vi "Master Control Loops Old.vi"() -> ()   [LabVIEW 2013]
uses:
  lib/DAQ IO/Daq Actions.ctl
  lib/Data Access Objects/Metadata/LBCB Number.ctl
  lib/Control Loop/Parameters Changes.ctl
  lib/Data Access Objects/Metadata/Persistant DAO Actions.ctl
  lib/MixedMode/Mixed Mode States.ctl
  lib/MixedMode/Ramp Time Tuple.ctl
  lib/MixedMode/Mixed Mode Command Action.ctl
  lib/MixedMode/Mixed Mode Convergence Status.ctl
  lib/MixedMode/Mixed Mode Cartesian Data.ctl
  lib/MixedMode/Target Data.ctl
  lib/MixedMode/Messages/Mixed Mode Command.ctl
  lib/Control Loop/Mixed Mode Hold Data type.ctl
  lib/Control Loop/Control Loop State.ctl
  lib/Data Access Objects/Metadata/DAO Actions.ctl
  lib/Control Loop/Parameter Change States.ctl
  lib/MixedMode/Messages/Mixed Mode Status.ctl
  lib/Apps/App Status Actions.ctl
  lib/Logging/LogFileType.ctl
  lib/Launcher/Launcher Actions.ctl
  lib/Launcher/NoPanelAppTypes.ctl
  lib/Autobalance/Autobalance State.ctl
  lib/Apps/Yes No Button.ctl
  lib/Control Loop/Limit Settings.ctl
  lib/Control Loop/Limit Matrix.ctl
  lib/Data Access Objects/Global Cache/Global Cache.vi
  lib/Control Loop/MM Result Actions.ctl
  lib/MixedMode/Stiffness Matrix.ctl
  lib/Limits/Cart Disp Faults.ctl
  lib/Limits/Cart Force Faults.ctl
  lib/Limits/Actuator Faults.ctl
  lib/Control Loop/Act & Cart Commands.ctl
  lib/Limits/Within Limits Matrix.ctl
  lib/Global Data/Jacobian Stiffness Column Id.ctl
  lib/Global Data/Jacobian Stiffness Column.ctl
  lib/Global Data/Dataset Source.ctl
  lib/Logging/Command or Stiffness Updates.ctl
  lib/Control Loop/Command Or Stiffness Update Type.ctl
  lib/Data Access Objects/Control Loop/PID Controls.ctl
  lib/Autobalance/Autobalance Status Data.ctl
  lib/Autobalance/Autobalance Stage.ctl
  lib/Autobalance/Autobalance Data Point.ctl
  lib/Control Loop/Measurements.ctl
  lib/Data Access Objects/Autobalance/Autobalance Control Parameters.ctl
panel:
  out "MM Result Actions":T1
  out "Commands":T2[](array[typedef])
  out "Stiffness Jacobian Column":T3[](array[typedef])
  out "Target":T5[](array[typedef])
  out "Cart Individual Cmds":dbl[][](array[numeric])=[[0.015224103858920254, 0.016374115079328375, 0.0001743188568230551, 0.03971045114557009, 0.007082336209989981, 0.009859079687370698, 8.685887933911959, 1.9897804119684945, 4.857688782335148, 93.30834661628205, -5.911514458784602, -1.446477360303783]]
  in  "AB Parameters":T6={"Number of Samples"=0, "Delay After Cmd"=0, "Maximum Command"=0.0, "1/4 Linear Range"=0.5}
  out "Increment Limits":T2[](array[typedef])
  out "Hold Data":T7[](array[typedef])
  in  "L2 Ctrl Loop In Actuator":dbl[](array[numeric])
  out "Rigid Connection":bool
  out "Stiffness Limits":dbl[][][](array[numeric])
  out "L2 Autobalance Out":T8[](array[typedef])
  out "L2 Cmd  Volts":dbl[](array[numeric])
  out "L2 Ctrl Loop Out Actuator":dbl[](array[numeric])=[0.012801822908652838, 0.012801822908652838, 7.98290599846041e-06, 8.154359441903125e-06, 8.154359441903125e-06, 8.154359441903125e-06]
  in  "Monitor Loop Time":u32
  in  "Volts LVDT & LC":dbl[][](array[numeric])
  out "L1 Autobalance Out":T8[](array[typedef])
  out "Collecting DAQ Samples":bool
  out "DAQ Volts":dbl[](array[numeric])=[-5.059315779335383, -5.016629198362524, -5.097891313865665, -5.092890991738198, -5.1138932889519, -4.974194835814303, 0.24442110332308561, 0.2508540081873783, -0.00045656932832031883, -0.0010919008583725697, -0.001119467422792373, -0.001138029771633142, 0.051584220664617125, 0.05637080163747566, -0.0007913138656640637, 0.023009008261802286, -0.021593288951899364, 0.0027051641856972383, -5.059665406563526, -5.018353952939143, -5.097893414204858, -5.0928919356893525, -5.11389113151188, -4.974191443340161, 0.24267296718237016, 0.2422302353042843, -0.0004670710242903981, -0.0011032282722249686, -0.0010935781425555466, -0.0010973200819313358, 0.05123459343647403, 0.05464604706085686, -0.0007934142048580796, 0.02300806431064792, -0.02159113151187963, 0.0027085566598390553, 0.048884220664617124, 0.04853459343647403, 0.050170801637475664, 0.04844604706085686, -9.131386566406377e-05, -9.341420485807962e-05]
  in  "Volt Logger Time":u32
  out "All Stopped":bool
  out "Previous Target":T12[](array[typedef])
  out "Iterative Target":T5[](array[typedef])
  out "Mixed Mode":i32
  out "Status Changes":i32
  out "L2 Control Rate":i32
  out "DAQ Started":bool
  out "Current Target":T5[](array[typedef])
  out "Logging Directory":path
  out "Auto Balance Error Tolerance":dbl[][](array[numeric])=[[0.01, 0.01, 0.01, 0.01, 0.01, 0.01]]
  in  "Hold Period":bool
  in  "Averaging":bool
  out "L1 Ctrl Loop State":T13
  out "Max Increment":dbl[][](array[numeric])
  out "Jacobian Gain":dbl[][](array[numeric])
  out "Force Error Range":dbl[][](array[numeric])
  in  "L2 PID On":bool
  in  "Limits Check":T14[](array[typedef])
  in  "Ramp Time":u32
  out "Limits":T18[](array[typedef])
  out "Measurements":T20[](array[typedef])
  out "Stiffness Jacobian":cluster{T21}[](array[cluster])
  out "Convergence Status":T22[](array[typedef])
  out "MixedModeStates":T23
  out "PID Control":T24[](array[typedef])
  in  "L1 PID On":bool
  out "LBCB 1 Control Loop Force Limit":bool
  out "L2 Ctrl Loop State":T13
  out "L1 Cmd  Volts":dbl[](array[numeric])
  out "L1 Ctrl Loop Out Actuator":dbl[](array[numeric])=[0.012801822908652838, 0.012801822908652838, 7.98290599846041e-06, 8.154359441903125e-06, 8.154359441903125e-06, 8.154359441903125e-06]
  out "L1 Control Rate":i32=50 caption="Control Rate"
  in  "L1 Ctrl Loop In Actuator":dbl[](array[numeric])
  out "Number of \nExternal \nChannels":i32
  out "DAQ Enabled":bool
  in  "App Running":bool
  out "DAQ Rate":i32=2 caption="Control Rate"
  out "Servo Error":dbl[][](array[numeric])=[[-0.014471871278962644, -0.0027477897622864888, 0.03594582291831433, -0.006177356244415369, -0.000527948512754489, 0.04718526152757189]]
  out "Actuator Meas. Disp & Forces":dbl[][](array[numeric])=[[0.015224103858920254, 0.016374115079328375, 0.0001743188568230551, 0.03971045114557009, 0.007082336209989981, 0.009859079687370698, 8.685887933911959, 1.9897804119684945, 4.857688782335148, 93.30834661628205, -5.911514458784602, -1.446477360303783]]
  out "External Sensors":dbl[](array[numeric])
  out "DAQ Overflow":bool
  # "(Volts)"
  # "Cmd"
  # "Servo"
  # "Cmd"
  # "Servo"
  # "Cmd"
  # "Servo"
  # "Cmd"
  # "Servo"
  # "Continuous"
  # "Hold"
types:
  T1 = typedef "MM Result Actions.ctl" = enum16{"Nop", "Set Command", "Check Limits", "Send Command", "Store Prev Reading", "Averaging On", "Averaging Off", "Hold On", "Hold Off", "PID Hold On", "PID Hold Off", "Clear Increment Faults", "Set Initial Position"}
  T2 = typedef "Act & Cart Commands.ctl" = cluster{"Act Cmd":dbl[], "Cart Cmd":dbl[]}
  T3 = typedef "Jacobian Stiffness Column.ctl" = cluster{"Id":T4, "Column":dbl[]}
  T4 = typedef "Jacobian Stiffness Column Id.ctl" = enum16{"dDx", "dDy", "dDz", "dRx", "dRy", "dRz"}
  T5 = typedef "Target Data.ctl" = cluster{"Displacements":dbl[], "Command Type":enum16{"<None>", "Displacement", "Force"}[], "Forces":dbl[]}
  T6 = typedef "Autobalance Control Parameters.ctl" = cluster{"Number of Samples":i32, "Delay After Cmd":i32, "Maximum Command":dbl, "1/4 Linear Range":dbl}
  T7 = typedef "Mixed Mode Hold Data type.ctl" = cluster{"Displacements":dbl[], "Forces":dbl[], "Displacement \nCommands":dbl[]}
  T8 = typedef "Autobalance Status Data.ctl" = cluster{"IsBalanced":T9, "Autobalance Stage":T10, "High":T11, "Low":T11, "Balanced \nCmd":dbl}
  T9 = typedef "Yes No Button.ctl" = bool
  T10 = typedef "Autobalance Stage.ctl" = enum16{"Coarse", "Fine", "Backing Up", "Done"}
  T11 = typedef "Autobalance Data Point.ctl" = cluster{"cCmd":dbl, "cServo":dbl, "pCmd":dbl, "pServo":dbl}
  T12 = typedef "Mixed Mode Cartesian Data.ctl" = cluster{"Displacements":dbl[], "Forces":dbl[]}
  T13 = typedef "Control Loop State.ctl" = enum16{"Idle", "Off", "Reset Autobalancing", "Autobalancing", "Set Command", "Ready for Control", "On"}
  T14 = typedef "Within Limits Matrix.ctl" = cluster{"Act Disp":T15, "Act Force":T15, "Act Incr":T15, "Cart Disp":T16, "Cart Force":T17, "Cart Incr":T16}
  T15 = typedef "Actuator Faults.ctl" = cluster{"X1":bool, "X2":bool, "Y1":bool, "Z1":bool, "Z2":bool, "Z3":bool}
  T16 = typedef "Cart Disp Faults.ctl" = cluster{"Dx":bool, "Dy":bool, "Dz":bool, "Rx":bool, "Ry":bool, "Rz":bool}
  T17 = typedef "Cart Force Faults.ctl" = cluster{"Fx":bool, "Fy":bool, "Fz":bool, "Mx":bool, "My":bool, "Mz":bool}
  T18 = typedef "Limit Settings.ctl" = cluster{"Actuator Force Limits":T19, "Actuator Stroke Limits":T19, "Cartesian Disp Limit":T19, "Cartesian Force Limit":T19}
  T19 = typedef "Limit Matrix.ctl" = dbl[][]
  T20 = typedef "Measurements.ctl" = cluster{"Act Disp":dbl[], "Act Forces":dbl[], "Cart Disp":dbl[], "Cart Forces":dbl[]}
  T21 = typedef "Stiffness Matrix.ctl" = dbl[][]
  T22 = typedef "Mixed Mode Convergence Status.ctl" = cluster{"IsConverged":bool[], "Force Errors":dbl[], "Controlling DOF":bool[]}
  T23 = typedef "Mixed Mode States.ctl" = enum16{"Init", "Wait For DAQ", "Idle", "Start Initial Position", "Initial Position", "Start Initial Ramp", "Run Initial Ramp", "Start Iterative Stage", "Convergence Check", "Update Stiffness Jacobian", "Update Command", "Start Iterative Ramp", "Run Iterative Ramp", "Start Iterative Stabilize", "Iterative Stabilize", "Start Iterative Holding", "Iterative Holding", "Start Stabilize", "Stabilize", "Start Hold", "Holding", "Done", "Aborting", "Exit", "Nop"}
  T24 = typedef "PID Controls.ctl" = cluster{"I-Control":bool, "Ctrl Mode":bool}
  T25 = typedef "Command Or Stiffness Update Type.ctl" = cluster{"Target":T5[], "Stiffness":T3[], "Command || Stiffness Update":T26}
  T26 = typedef "Command or Stiffness Updates.ctl" = enum16{"Command Update", "Iterative Command Update", "Stiffness Update"}
  T27 = cluster{"Act Disp":dbl[], "Act Forces":dbl[], "Cart Disp":dbl[], "Cart Forces":dbl[]}
  T28 = typedef "LBCB Number.ctl" = enum16{"LBCB1", "LBCB2"}
  T29 = typedef "Persistant DAO Actions.ctl" = enum16{"Init", "Get", "Set", "Load", "Save"}
  T30 = typedef "Autobalance State.ctl" = enum16{"Init", "Send High ", "Wait High", "Read High Start", "Read High", "Send Low", "Wait Low", "Read Low Start", "Read Low", "Publish", "Calculate", "Done"}
  T31 = typedef "Ramp Time Tuple.ctl" = cluster{"Ramp":dbl, "Stab":dbl, "Hold":dbl}
  T32 = typedef "Mixed Mode Command Action.ctl" = enum16{"Start Command", "Stop", "Exit", "No Op", "Start Acquisition", "Measure Initial Position"}
  T33 = typedef "Mixed Mode Status.ctl" = cluster{"LBCB Target":T5[], "MixedModeStates":T23, "LBCB Convergence":T22[], "LBCB Measurements":T12[]}
  T34 = typedef "Mixed Mode Command.ctl" = cluster{"Command":T32, "Ramp Times":cluster{"Initial":T31, "Iterative":T31}, "LBCB1":T5, "LBCB2":T5}
  T35 = typedef "Parameters Changes.ctl" = cluster{"Change State":T36, "LBCB Number":T28}
  T36 = typedef "Parameter Change States.ctl" = enum16{"Mixed Mode", "Control Loop", "Limits", "Application", "Stiffness Jacobian", "Start DAQ", "Reset Auto-Balance", "Set Command", "Enable Control", "Disable Control", "Position", "Stop Application"}
  T37 = typedef "DAO Actions.ctl" = enum16{"Init", "Get", "Set"}
  T38 = typedef "Number Of LBCBs.ctl" = enum16{"1", "2"}
  T39 = typedef "Cartesian Point.ctl" = cluster{"Dx":dbl, "Dy":dbl, "Dz":dbl, "Rx":dbl, "Ry":dbl, "Rz":dbl}
  T40 = typedef "Actuator Matrix.ctl" = cluster{"Lower":T41, "Upper":T41}
  T41 = typedef "Actuator Point.ctl" = cluster{"X1":dbl, "X2":dbl, "Y1":dbl, "Z1":dbl, "Z2":dbl, "Z3":dbl}
  T42 = typedef "Cartesian Matrix.ctl" = cluster{"Lower":T39, "Upper":T39}
  T43 = typedef "App Parameters.ctl" = cluster{"Monitor Loop":T44, "Ramp Time":T44, "Log Loop":T44, "TCP to DAQ":T44, "Logging Directory":path, "Log File Size (MBytes)":i64, "Volt Logging Loop":T44, "2 LBCB Archiving Mode":bool, "Fake":bool}
  T44 = typedef "Timing Parameters.ctl" = cluster{"Interval":dbl, "Rate ":dbl}
  T45 = typedef "Dataset Source.ctl" = enum16{"Continuous", "Hold", "ED", "Volts", "Offsets", "Increments"}
  T46 = typedef "Calibration Settings.ctl" = cluster{"Command Sensitivity":dbl[], "Servo Error Offset":dbl[], "LVDT Sensitivity":dbl[], "LVDT Offset":dbl[], "Load Cell Offsets":dbl[], "Load Cell Sensitivity":dbl[]}
  T47 = typedef "App Status Actions.ctl" = enum16{"Init", "Get Status", "Running", "Control", "Autobalanced", "Data Acquisition", "Set App State", "DAQ Started", "Set LBCB State", "Set All", "Set Cont Logging", "Set Step Logging", "Set MM Logging", "Set Volt Logging", "Set DAQ Link"}
  T48 = typedef "Force Control Parameters.ctl" = cluster{"Use Force Error Range Ratios":bool, "Use Group Priorities":bool, "Multi Command Update":bool, "Steps per Stiffness \nMeasurement":i32}
  T49 = typedef "Cartesian Force Vector.ctl" = cluster{"Fx":dbl, "Fy":dbl, "Fz":dbl, "Mx":dbl, "My":dbl, "Mz":dbl}
  T50 = typedef "Ramp Time Input.ctl" = cluster{"Directional":T51, "Iterative":T51}
  T51 = typedef "Ramp Control.ctl" = cluster{"Ramp":dbl, "Stabilize":dbl, "Hold":dbl}
  T52 = typedef "App Status.ctl" = cluster{"Running":bool, "Controlling L2":bool, "Autobalance L2":bool, "Data Acquisition":bool, " App State":T53, "DAQ Started":bool, "LBCB 1 State":T54, "LBCB 2 State":T54, "Controlling L1":bool, "Autobalance L1":bool, "Continuous Logging":bool, "Step Logging":bool, "Voltage Logging":bool, "Mixed Mode Logging":bool, "DAQ Link":bool}
  T53 = typedef "AppStates.ctl" = enum16{"Starting OM", "Initializing Displays", "Setting up Archiving", "Setting Up DAQ Channels", "Start DAQ", "DAQ Starting", "Controlling LBCBs", "Stopping OM"}
  T54 = typedef "Lbcb Control Loop States.ctl" = enum16{"Idle", "Start Selected", "Load Last Command", "Start Autobalancing", "Autobalancing", "Control Loop Initialized", "Control Enabled"}
  T55 = cluster{"Act Disp":dbl[], "Act Forces":dbl[], "Cart Disp":dbl[], "Cart Forces":dbl[]}[]
  T56 = typedef "Daq Actions.ctl" = enum16{"Init", "Send Commands", "Get Responses", "Stop"}
  T57 = enum16{"open", "replace", "create", "open or create", "replace or create", "replace or create with confirmation"}
  T58 = typedef "LogFileType.ctl" = enum16{"Continuous", "Step", "Volts", "Offsets", "DLL  Errors", "Snapshot", "Commands", "StiffnessUpdates", "Debug", "End List"}
  T59 = typedef "NoPanelAppTypes.ctl" = enum16{"NTCP Socket", "Data Archiving", "DAQ Link", "Control Loops", "Cmd Disp Diffs", "LBCB Data", "Limits", "Mixed Mode Widget", "Offsets", "Debug"}
  T60 = typedef "Launcher Actions.ctl" = enum16{"Launch", "Stop All", "Stop", "Kill", "Running?", "Init"}
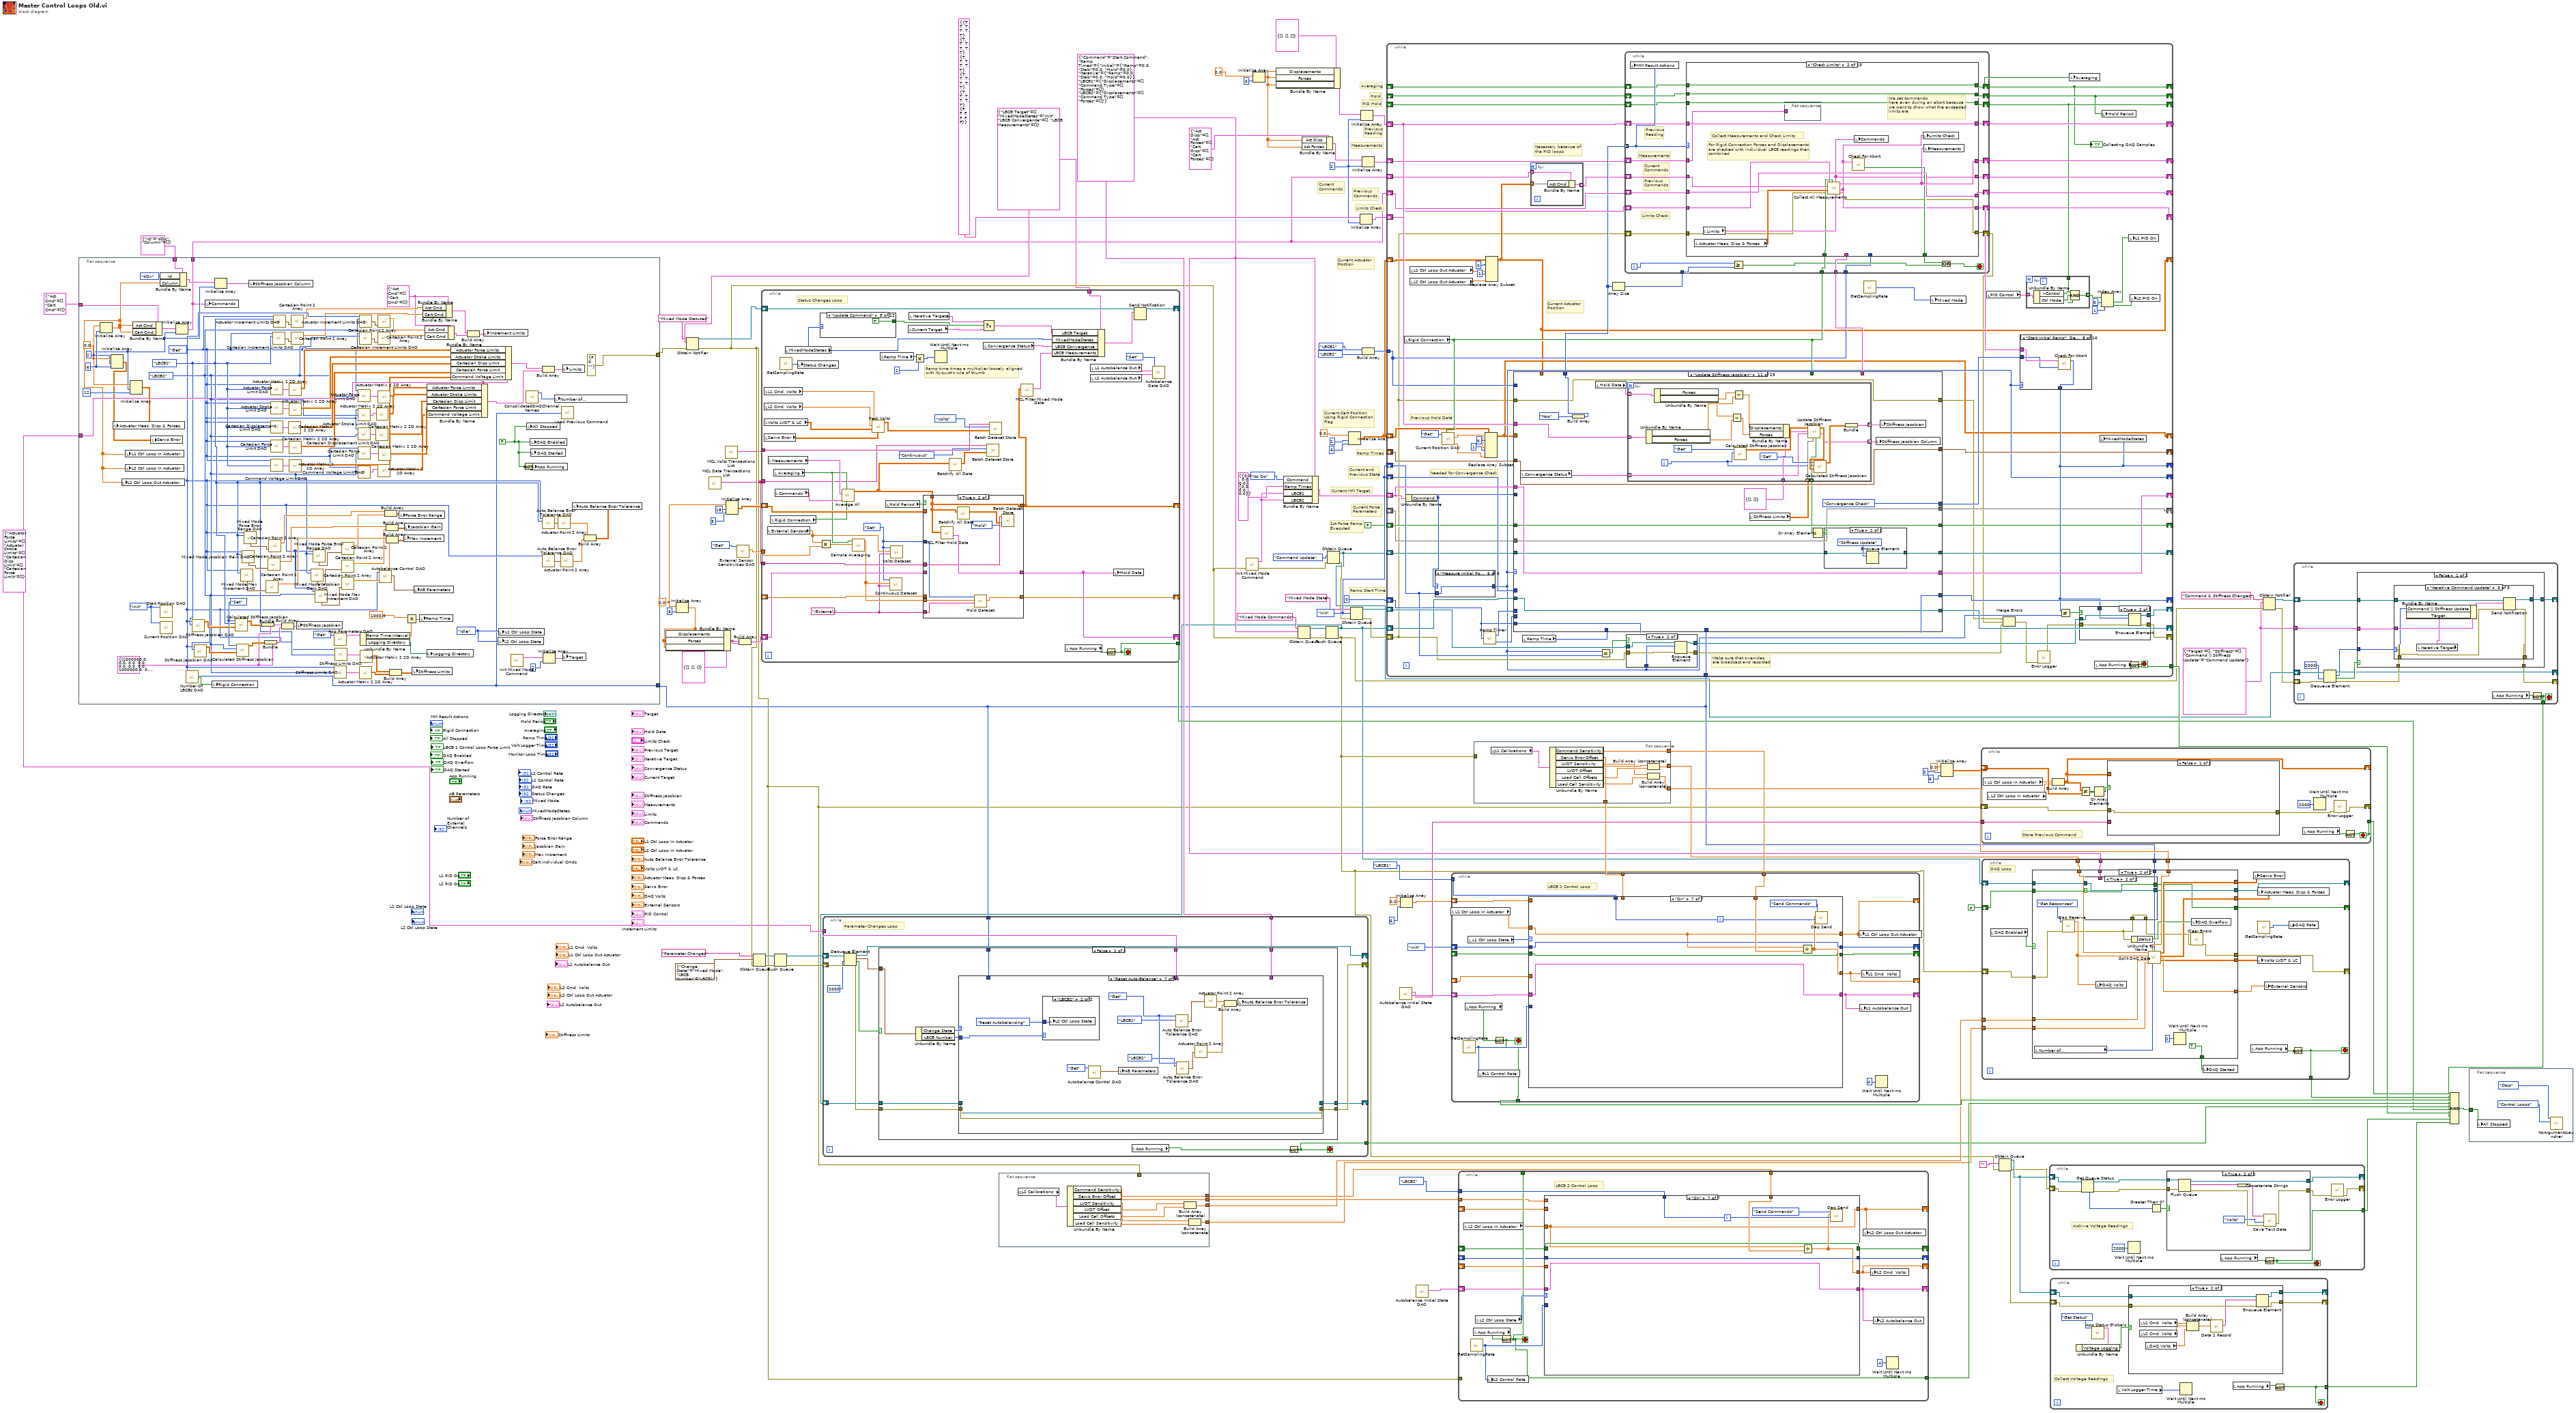
[diagram p0: block diagram]
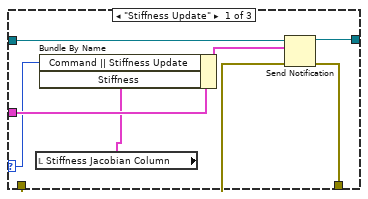
[diagram p2: hidden frame]
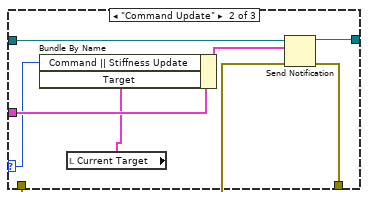
[diagram p3: hidden frame]
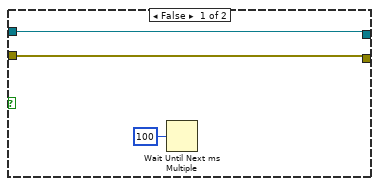
[diagram p5: hidden frame]
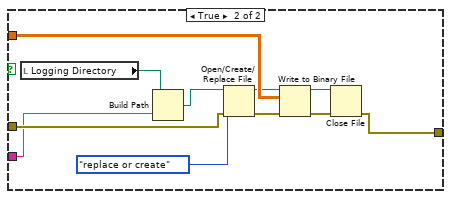
[diagram p7: hidden frame]
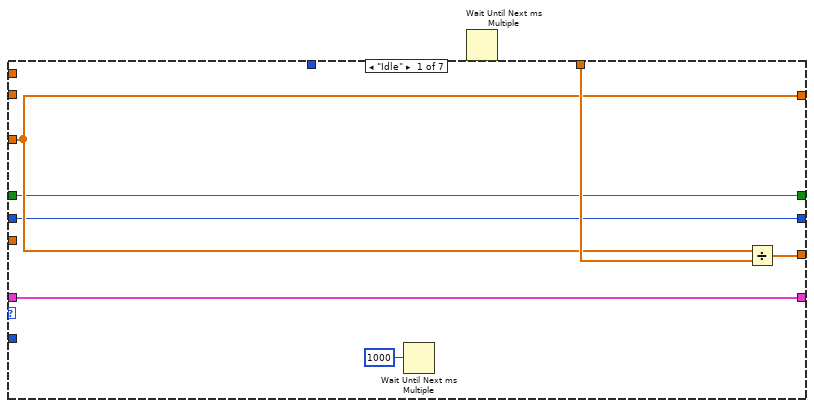
[diagram p8: hidden frame]
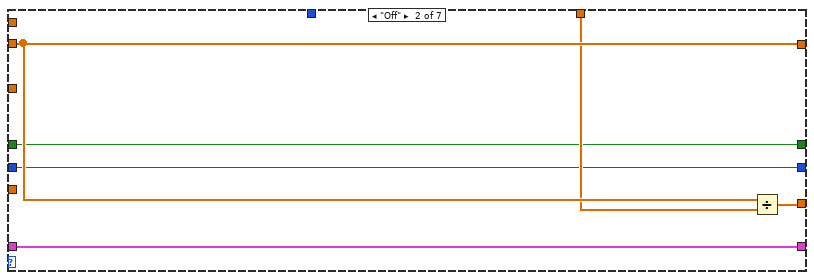
[diagram p9: hidden frame]
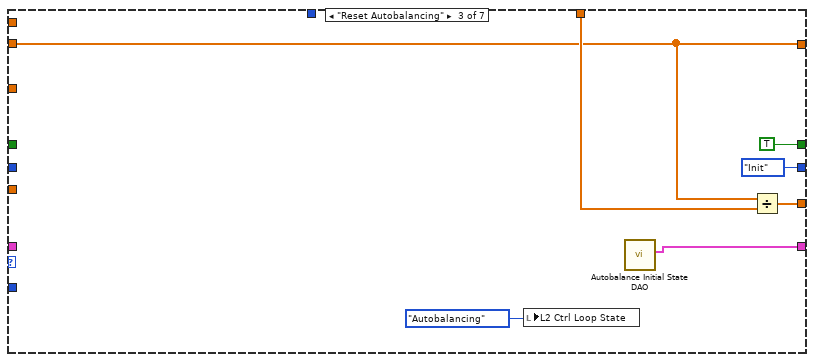
[diagram p10: hidden frame]
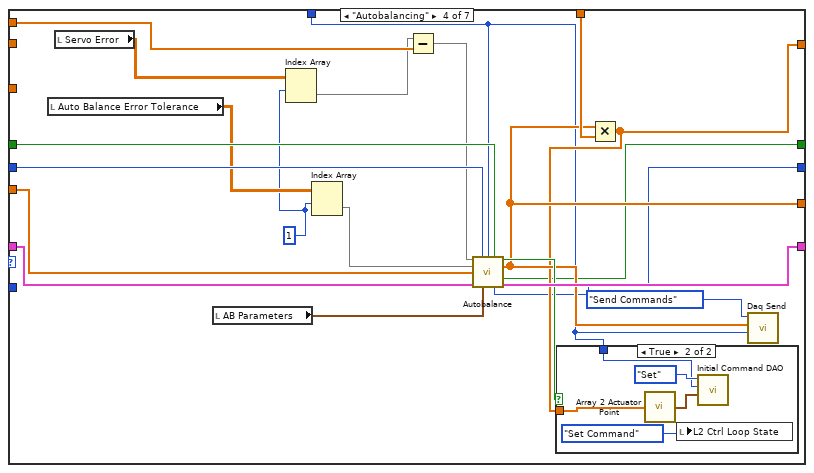
[diagram p11: hidden frame]
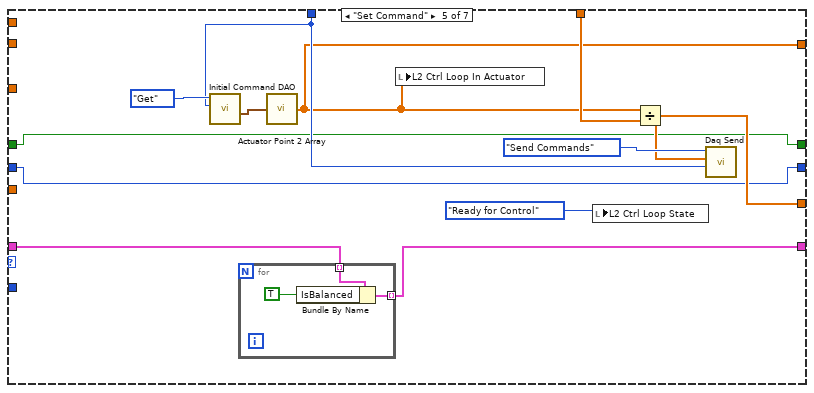
[diagram p13: hidden frame]
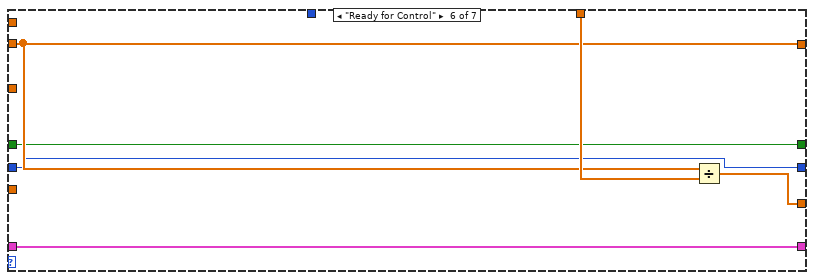
[diagram p14: hidden frame]
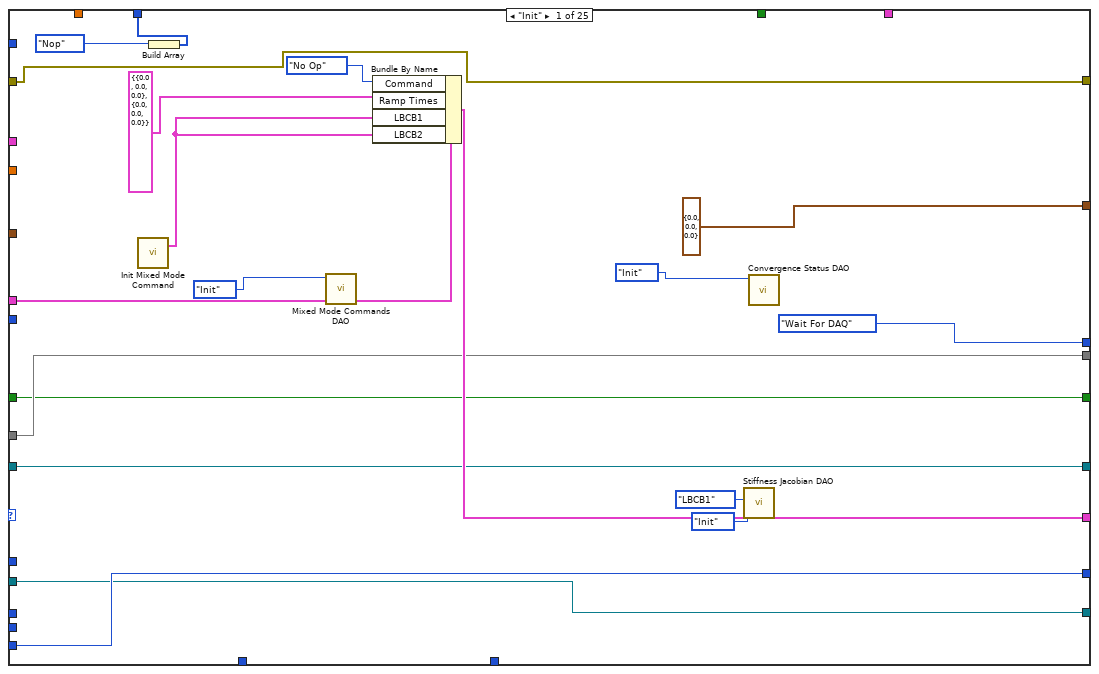
[diagram p15: hidden frame]
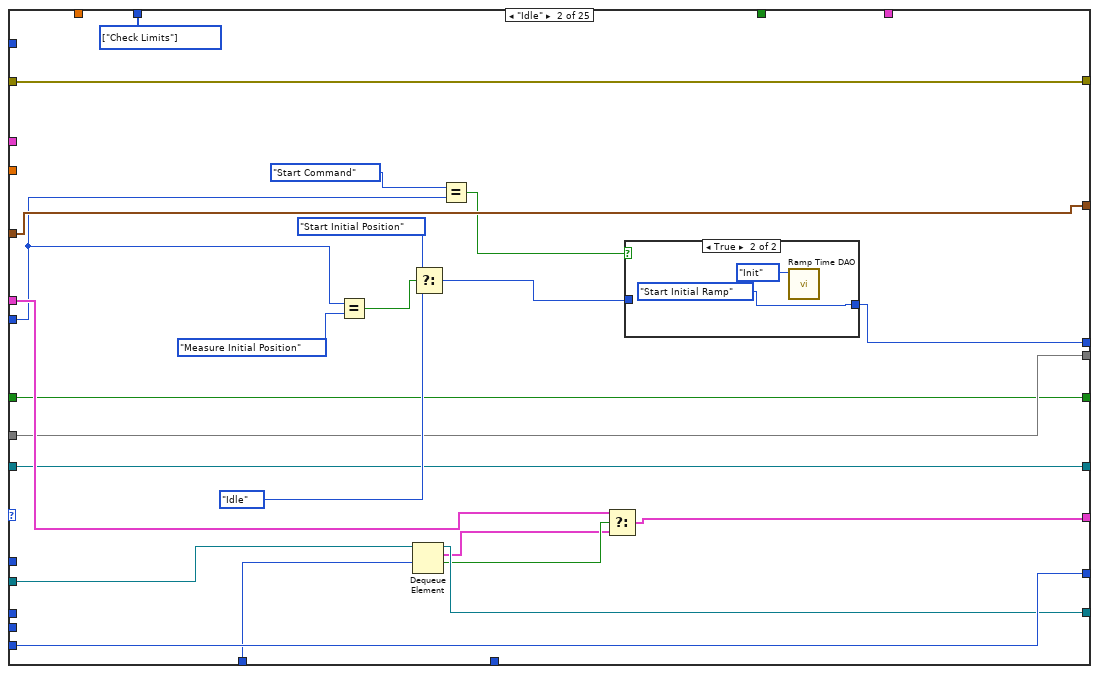
[diagram p16: hidden frame]
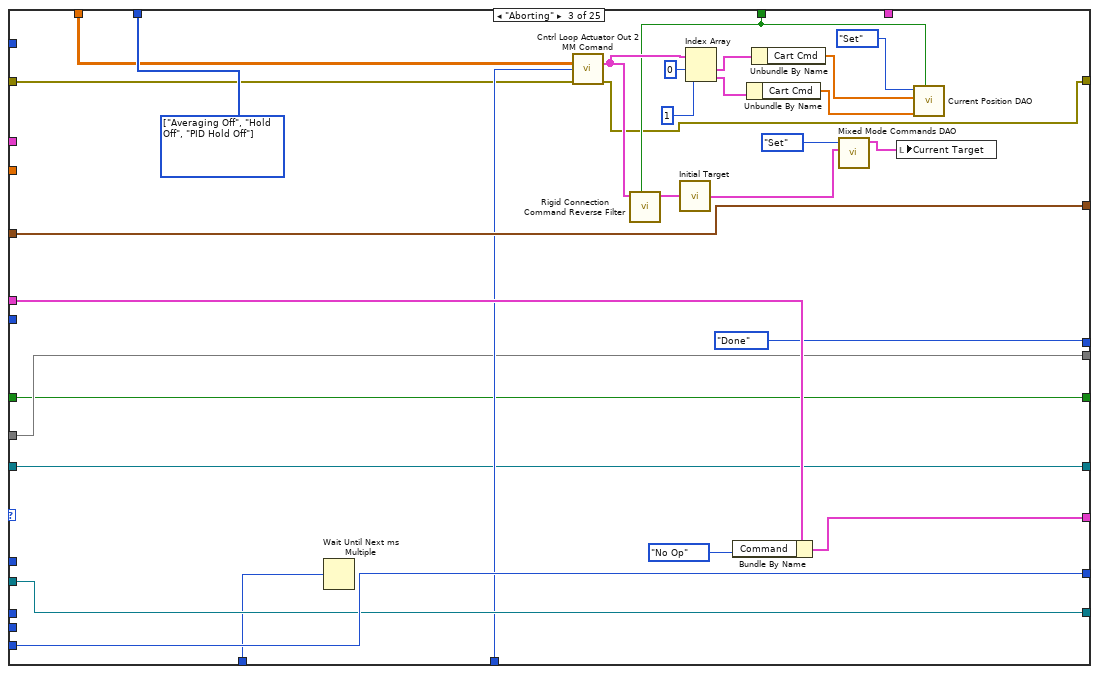
[diagram p18: hidden frame]
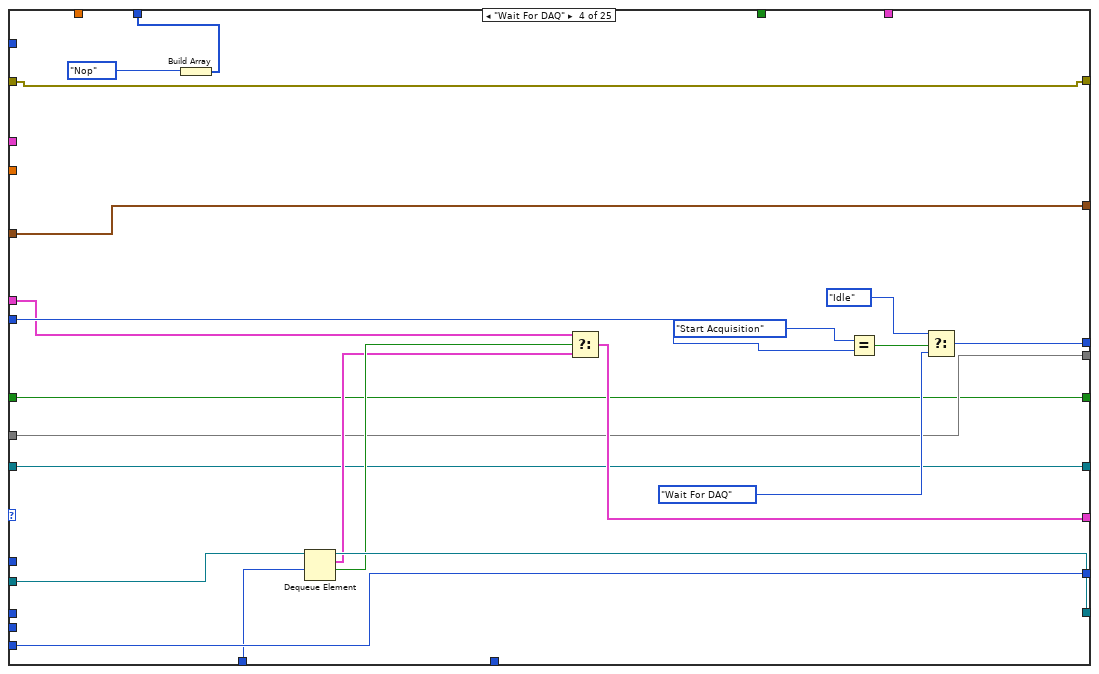
[diagram p19: hidden frame]
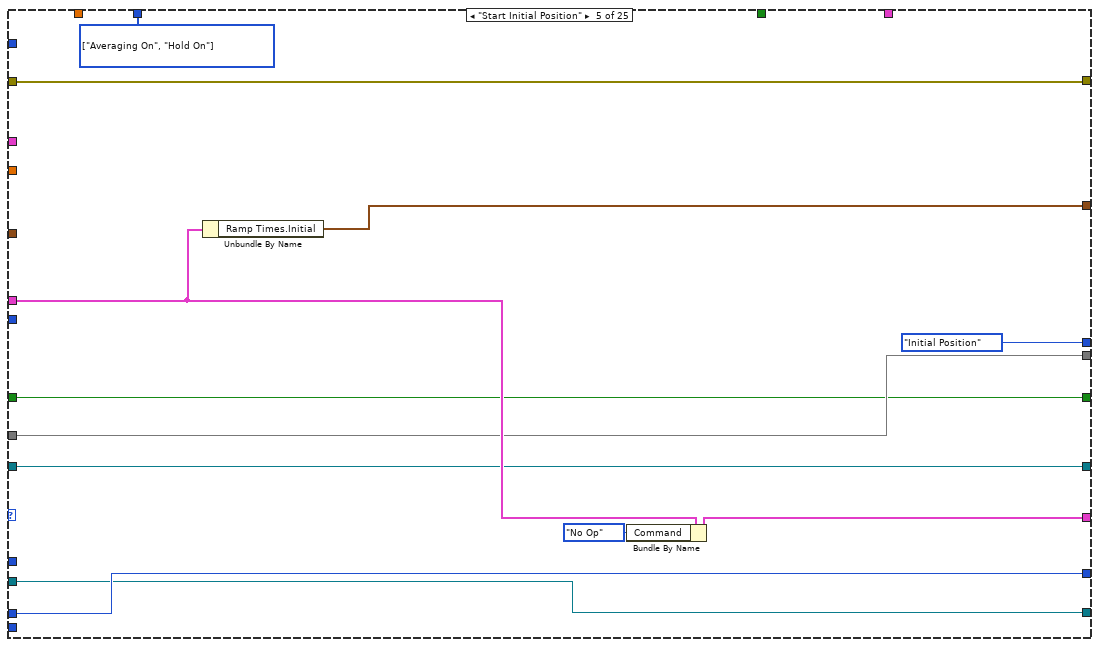
[diagram p20: hidden frame]
diagram:
  w7 = T25 {"Target"=[], "Stiffness"=[], "Command || Stiffness Update"=enum."Command Update"} ("Command || Stiffness Update")
  w18 = 0.0 ("element")
  w38 = 2 ("dimension size")
  w59 = T18 {"Actuator Force Limits"=[], "Actuator Stroke Limits"=[], "Cartesian Disp Limit"=[], "Cartesian Force Limit"=[]} ("L1  Limits")
  w97 = T33 {"LBCB Target"=[], "MixedModeStates"=enum."Init", "LBCB Convergence"=[], "LBCB Measurements"=[]} ("Mixed Mode Status")
  w57 = T34 {"Command"=enum."Start Command", "Ramp Times"={"Initial"={"Ramp"=0.0, "Stab"=0.0, "Hold"=0.0}, "Iterative"={"Ramp"=0.0, "Stab"=0.0, "Hold"=0.0}}, "LBCB1"={"Displacements"=[], "Command Type"=[], "Forces"=[]}, "LBCB2"={"Displacements"=[], "Command Type"=[], "Forces"=[]}} ("Mixed Mode Command")
  w104 = Mixed_Mode_States."Init" ("MixedModeStates")
  # "Current Actuator\nPostion"
  # "Current Cart Position\nUsing Rigid Connection\nFlag"
  # "1st Force Ramp\nExecuted"
  # "Current Force\nParameters"
  # "Previous\nCommands"
  # "Limits Check"
  # "Ramp Start Time"
  # "PID Hold"
  # "Hold"
  # "Averaging"
  # "Previous\nReading"
  # "Current \nCommands"
  # "Measurements"
  # "Current MM Target"
  # "Current and\nPrevious State"
  # "Ramp Times"
  n1 = flat-sequence {
    tunnel: [errorcluster {"status"=FALSE, "code"=0, "source"=""} ("error out")] -> w62
    tunnel: w59 -> [w188]
    tunnel: [w109] -> w39
    tunnel: [w112] -> w37
    tunnel: T3 {"Id"=enum."dDx", "Column"=[]} ("Jacobian Stiffness Column") -> [w121]
    tunnel: T2 {"Act Cmd"=[], "Cart Cmd"=[]} ("Data") -> [w116]
    frame #0 {
      w123 = DAO_Actions."Init" ("DAO Actions")
      w125 = T2 {"Act Cmd"=[], "Cart Cmd"=[]} ("Data")
      w156 = cluster{T21} {[[1000000.0, 0.0, 0.0, 0.0, 0.0, 0.0], [0.0, 1000000.0, 0.0, 0.0, 0.0, 0.0], [0.0, 0.0, 1000000.0, 0.0, 0.0, 0.0], [0.0, 0.0, 0.0, 1000000.0, 0.0, 0.0], [0.0, 0.0, 0.0, 0.0, 1000000.0, 0.0], [0.0, 0.0, 0.0, 0.0, 0.0, 1000000.0]]} ("Cluster")
      w122 = 2 ("dimension size")
      w190 = Control_Loop_State."Idle" ("L1 Ctrl Loop State")
      w160 = 6 ("dimension size")
      w159 = 0.0 ("element")
      w133 = LBCB_Number."LBCB2" ("ID")
      w134 = LBCB_Number."LBCB1" ("ID")
      w132 = Persistant_DAO_Actions."Get" ("Actuator Force Limit Actions")
      w194 = FALSE
      w200 = Persistant_DAO_Actions."Set" ("Actions")
      n2 = Initialize Array(w159, w160) -> (w119:dbl[])
      n3 = Initialize Array(w159, w122, w160) -> (w137:dbl[][])
      n4 = local write "L1 Ctrl Loop Out Actuator"(w119) -> ()
      n5 = local write "L1 Ctrl Loop In Actuator"(w119) -> ()
      n6 = local write "L2 Ctrl Loop In Actuator"(w119) -> ()
      n7 = Initialize Array(w159, w122, 12 ("dimension size")) -> (w124:dbl[][])
      n8 = local write "Actuator Meas. Disp & Forces"(w124) -> ()
      n9 = Bundle By Name(cluster=w116, "Act Cmd"=w119, "Cart Cmd"=w119) -> (w142:T2)
      n10 = local write "Servo Error"(w137) -> ()
      n11 = call "Start Position DAO.vi"("DAO Actions"=w123) -> ()  [unwired: 9 in, 2 out]
      n12 = call "Current Position DAO.vi"("Actions"=w123) -> ()  [unwired: 9 in, 2 out]
      n13 = Bundle By Name(cluster=w121, "Id"=Jacobian_Stiffness_Column_Id."dDx", "Column"=w119) -> (w118:T3)
      n14 = Initialize Array(w142, w122) -> (w112:T2[])
      n15 = call "Number Of LBCBs DAO.vi"("Actions"=w132) -> ("Number of\nLBCBs Out"=w109:T38, "Rigid Connection Out"=w143:bool)  [unwired: 13 in, 4 out]
      n16 = call "Stiffness Jacobian DAO.vi"("LBCB Number"=w134, "Actions"=w132) -> ("Stiffness Jacobian Out"=w199:T21)  [unwired: 3 in, 6 out]
      n17 = call "Stiffness Jacobian DAO.vi"("LBCB Number"=w133, "Actions"=w132) -> ("Stiffness Jacobian Out"=w201:T21)  [unwired: 3 in, 6 out]
      n18 = local write "Commands"(w112) -> ()
      n19 = local write "Rigid Connection"(w143) -> ()
      n20 = Initialize Array(w118, w122) -> (w117:T3[])
      n21 = call "Calculated Stiffness Jacobian.vi"("Stiffness Jacobian In"=w199, "LBCB Number"=w134, "Actions"=w200) -> ("Stiffness Jacobian Out"=w158:T21)  [unwired: 1 in, 7 out]
      n22 = call "Calculated Stiffness Jacobian.vi"("Stiffness Jacobian In"=w201, "LBCB Number"=w133, "Actions"=w200) -> ("Stiffness Jacobian Out"=w157:T21)  [unwired: 1 in, 7 out]
      n23 = call "Mixed Mode Max Increment DAO.vi"("Max Increment Actions"=w132, "LBCB Number"=w134) -> ("Max Increment Out"=w207:T39)  [unwired: 3 in, 10 out]
      n24 = call "Mixed Mode Jacobian Gain DAO.vi"("Jacobian Gain Actions"=w132, "LBCB Number"=w134) -> ("Jacobian Gain Out"=w206:T39)  [unwired: 3 in, 10 out]
      n25 = call "Mixed Mode Force Error Range DAO.vi"("Force Error Range Actions"=w132, "LBCB Number"=w134) -> ("Force Error Range Out"=w205:T39)  [unwired: 3 in, 10 out]
      n26 = local write "Stiffness Jacobian Column"(w117) -> ()
      n27 = Bundle(cluster=w156, w158) -> (w155:cluster{T21})
      n28 = Bundle(cluster=w156, w157) -> (w154:cluster{T21})
      n29 = call "Cartesian Point 2 Array.vi"("Cart Disp"=w207) -> ("Array"=w202:dbl[])  [unwired: 2 out]
      n30 = call "Cartesian Point 2 Array.vi"("Cart Disp"=w206) -> ("Array"=w203:dbl[])  [unwired: 2 out]
      n31 = call "Cartesian Point 2 Array.vi"("Cart Disp"=w205) -> ("Array"=w204:dbl[])  [unwired: 2 out]
      n32 = call "Actuator Force Limit DAO.vi"("Actuator Force Limit Actions"=w132, "ID"=w134) -> ("Actuator Force Limits Out"=w187:T40)  [unwired: 3 in, 10 out]
      n33 = call "Actuator Stroke Limit DAO.vi"("Actuator Stroke Limit Actions"=w132, "ID"=w134) -> ("Actuator Stroke Limits Out"=w186:T40)  [unwired: 3 in, 10 out]
      n34 = call "Cartesian Displacement Limit DAO.vi"("Cartesian Displacement Limit Actions"=w132, "ID"=w134) -> ("Cartesian Displacement Out"=w181:T42)  [unwired: 3 in, 10 out]
      n35 = call "Cartesian Force Limit DAO.vi"("Cartesian Force Limit Actions"=w132, "ID"=w134) -> ("Cartesian Force Limit Out"=w180:T42)  [unwired: 3 in, 10 out]
      n36 = call "Command Voltage Limit DAO.vi"("Actuator Stroke Limit Actions"=w132, "ID"=w134) -> ("Command Voltage Limit Out"=w185:T40)  [unwired: 3 in, 10 out]
      n37 = call "Cartesian Increment Limits DAO.vi"("Actions"=w132, "LBCB Number"=w134) -> ("Inc Limits Out"=w141:T39)  [unwired: 11 in, 2 out]
      n38 = call "Actuator Increment Limits DAO.vi"("Actions"=w132, "LBCB Number"=w134) -> ("Inc Limits Out"=w136:T41)  [unwired: 11 in, 2 out]
      n39 = Build Array(w155, w154) -> (w153:cluster{T21}[])
      n40 = call "Cartesian Matrix 2 2D Array.vi"("Matrix In"=w181) -> ("Matrix Out"=w169:T19)  [unwired: 10 out]
      n41 = call "Actuator Matrix 2 2D Array.vi"("Matrix In"=w187) -> ("Matrix Out"=w184:T19)  [unwired: 10 out]
      n42 = call "Actuator Matrix 2 2D Array.vi"("Matrix In"=w186) -> ("Matrix Out"=w183:T19)  [unwired: 10 out]
      n43 = call "Cartesian Matrix 2 2D Array.vi"("Matrix In"=w180) -> ("Matrix Out"=w168:T19)  [unwired: 10 out]
      n44 = call "Actuator Matrix 2 2D Array.vi"("Matrix In"=w185) -> ("Matrix Out"=w182:T19)  [unwired: 10 out]
      n45 = call "Cartesian Point 2 Array.vi"("Cart Disp"=w141) -> ("Array"=w129:dbl[])  [unwired: 2 in]
      n46 = call "Cartesian Point 2 Array.vi"("Cart Disp"=w136) -> ("Array"=w131:dbl[])  [unwired: 2 in]
      n47 = local write "Stiffness Jacobian"(w153) -> ()
      n48 = call "Mixed Mode Jacobian Gain DAO.vi"("Jacobian Gain Actions"=w132, "LBCB Number"=w133) -> ("Jacobian Gain Out"=w192:T39)  [unwired: 3 in, 10 out]
      n49 = call "Mixed Mode Force Error Range DAO.vi"("Force Error Range Actions"=w132, "LBCB Number"=w133) -> ("Force Error Range Out"=w191:T39)  [unwired: 3 in, 10 out]
      n50 = call "Mixed Mode Max Increment DAO.vi"("Max Increment Actions"=w132, "LBCB Number"=w133) -> ("Max Increment Out"=w193:T39)  [unwired: 3 in, 10 out]
      n51 = call "App Parameters DAO.vi"("Actions"=Persistant_DAO_Actions."Get") -> ("Application Timing and Logging Out"=w211:T43)  [unwired: 3 in, 7 out]
      n52 = call "Stiffness Limits DAO.vi"("Actions"=w132, "ID"=w133) -> ("Stiffness Limit Out"=w146:T42)  [unwired: 11 in, 2 out]
      n53 = call "Stiffness Limits DAO.vi"("Actions"=w132, "ID"=w134) -> ("Stiffness Limit Out"=w148:T42)  [unwired: 11 in, 2 out]
      n54 = call "Cartesian Point 2 Array.vi"("Cart Disp"=w191) -> ("Array"=w166:dbl[])  [unwired: 1 in, 1 out]
      n55 = call "Cartesian Point 2 Array.vi"("Cart Disp"=w192) -> ("Array"=w164:dbl[])  [unwired: 1 in, 1 out]
      n56 = call "Cartesian Point 2 Array.vi"("Cart Disp"=w193) -> ("Array"=w162:dbl[])  [unwired: 1 in, 1 out]
      n57 = call "Actuator Force Limit DAO.vi"("Actuator Force Limit Actions"=w132, "ID"=w133) -> ("Actuator Force Limits Out"=w179:T40)  [unwired: 3 in, 10 out]
      n58 = call "Actuator Stroke Limit DAO.vi"("Actuator Stroke Limit Actions"=w132, "ID"=w133) -> ("Actuator Stroke Limits Out"=w178:T40)  [unwired: 3 in, 10 out]
      n59 = call "Cartesian Displacement Limit DAO.vi"("Cartesian Displacement Limit Actions"=w132, "ID"=w133) -> ("Cartesian Displacement Out"=w177:T42)  [unwired: 3 in, 10 out]
      n60 = call "Cartesian Force Limit DAO.vi"("Cartesian Force Limit Actions"=w132, "ID"=w133) -> ("Cartesian Force Limit Out"=w176:T42)  [unwired: 3 in, 10 out]
      n61 = call "Command Voltage Limit DAO.vi"("Actuator Stroke Limit Actions"=w132, "ID"=w133) -> ("Command Voltage Limit Out"=w175:T40)  [unwired: 3 in, 10 out]
      n62 = call "Cartesian Increment Limits DAO.vi"("Actions"=w132, "LBCB Number"=w133) -> ("Inc Limits Out"=w140:T39)  [unwired: 11 in, 2 out]
      n63 = call "Actuator Increment Limits DAO.vi"("Actions"=w132, "LBCB Number"=w133) -> ("Inc Limits Out"=w135:T41)  [unwired: 11 in, 2 out]
      n64 = call "Actuator Matrix 2 2D Array.vi"("Matrix In"=w146) -> ("Matrix Out"=w145:T19)  [unwired: 10 out]
      n65 = Unbundle By Name(w211) -> ("Ramp Time.Interval"=w212:dbl, "Logging Directory"=w208:path)
      n66 = call "Actuator Matrix 2 2D Array.vi"("Matrix In"=w148) -> ("Matrix Out"=w147:T19)  [unwired: 10 out]
      n67 = call "Cartesian Matrix 2 2D Array.vi"("Matrix In"=w177) -> ("Matrix Out"=w172:T19)  [unwired: 10 out]
      n68 = call "Actuator Matrix 2 2D Array.vi"("Matrix In"=w178) -> ("Matrix Out"=w173:T19)  [unwired: 10 out]
      n69 = call "Cartesian Point 2 Array.vi"("Cart Disp"=w140) -> ("Array"=w128:dbl[])  [unwired: 2 in]
      n70 = call "Cartesian Point 2 Array.vi"("Cart Disp"=w135) -> ("Array"=w130:dbl[])  [unwired: 2 in]
      n71 = call "Actuator Matrix 2 2D Array.vi"("Matrix In"=w179) -> ("Matrix Out"=w174:T19)  [unwired: 10 out]
      n72 = call "Actuator Matrix 2 2D Array.vi"("Matrix In"=w175) -> ("Matrix Out"=w170:T19)  [unwired: 10 out]
      n73 = call "Cartesian Matrix 2 2D Array.vi"("Matrix In"=w176) -> ("Matrix Out"=w171:T19)  [unwired: 10 out]
      n74 = call "Autobalance Control DAO.vi"("Persistent DAO Actions"=w132) -> ("Autobalance Control Out"=w138:T6)  [unwired: 8 in, 2 out]
      n75 = Build Array(w204, w166) -> (w167:dbl[][])
      n76 = Build Array(w203, w164) -> (w165:dbl[][])
      n77 = Build Array(w202, w162) -> (w163:dbl[][])
      n78 = Build Array(w147, w145) -> (w144:dbl[][][])
      n79 = local write "Force Error Range"(w167) -> ()
      n80 = local write "Max Increment"(w163) -> ()
      n81 = local write "Jacobian Gain"(w165) -> ()
      n82 = Multiply(x=1000.0, y=w212) -> (x*y=w209:dbl)
      n83 = local write "Stiffness Limits"(w144) -> ()
      n84 = local write "AB Parameters"(w138) -> ()
      n85 = local write "Ramp Time"(w209) -> ()
      n86 = Bundle By Name(cluster=w125, "Act Cmd"=w131, "Cart Cmd"=w129) -> (w127:T2)
      n87 = Bundle By Name(cluster=w125, "Act Cmd"=w130, "Cart Cmd"=w128) -> (w126:T2)
      n88 = local write "Logging Directory"(w208) -> ()
      n89 = Bundle By Name(cluster=w188, "Actuator Force Limits"=w174, "Actuator Stroke Limits"=w173, "Cartesian Disp Limit"=w172, "Cartesian Force Limit"=w171, "Command Voltage Limit"=w170) -> (w149:T18)
      n90 = Bundle By Name(cluster=w188, "Actuator Force Limits"=w184, "Actuator Stroke Limits"=w183, "Cartesian Disp Limit"=w169, "Cartesian Force Limit"=w168, "Command Voltage Limit"=w182) -> (w189:T18)
      n91 = Build Array(w127, w126) -> (w139:T2[])
      n92 = local write "Increment Limits"(w139) -> ()
      n93 = local write "L2 Ctrl Loop State"(w190) -> ()
      n94 = local write "L1 Ctrl Loop State"(w190) -> ()
      n95 = call "Init Mixed Mode Command.vi"() -> ("Command Data"=w115:T5)  [unwired: 2 in, 1 out]
      n96 = Not(x=w194) -> (.not. x?=w198:bool)
      n97 = call "ConsolidatedDAQChannelNames.vi"() -> ("Number of \nExternal \nChannels 1"=w197:i32)  [unwired: 5 out]
      n98 = local write "All Stopped"(w194) -> ()
      n99 = local write "DAQ Enabled"(w194) -> ()
      n100 = local write "DAQ Started"(w194) -> ()
      n101 = local write "App Running"(w198) -> ()
      n102 = call "Auto Balance Error Tolerance DAO.vi"("Auto Balance Increment Actions"=w132, "LBCB Number"=w134) -> ("Auto Balance Error Out"=w111:T41)  [unwired: 3 in, 10 out]
      n103 = Build Array(w189, w149) -> (w150:T18[])
      n104 = call "Auto Balance Error Tolerance DAO.vi"("Auto Balance Increment Actions"=w132) -> ("Auto Balance Error Out"=w110:T41)  [unwired: 4 in, 10 out]
      n105 = Initialize Array(w115, 2 ("dimension size")) -> (w114:T5[])
      n106 = local write "Number of \nExternal \nChannels"(w197) -> ()
      n107 = call "Actuator Point 2 Array.vi"("Actuator Point"=w111) -> ("Array"=w196:dbl[])
      n108 = call "Actuator Point 2 Array.vi"("Actuator Point"=w110) -> ("Array"=w151:dbl[])
      n109 = call "Load Previous Command.vi"("Number of LBCBs"=w109) -> ()  [unwired: 3 out]
      n110 = local write "Limits"(w150) -> ()
      n111 = local write "Target"(w114) -> ()
      n112 = Build Array(w196, w151) -> (w152:dbl[][])
      n113 = local write "Auto Balance Error Tolerance"(w152) -> ()
    }
  }
  n114 = Initialize Array(w18, 6 ("dimension size")) -> (w35:dbl[])
  n115 = Bundle By Name(cluster=T7 {"Displacements"=[], "Forces"=[], "Displacement \nCommands"=[]} ("element"), "Displacements"=w35, "Forces"=w35, "Displacement \nCommands"=w35) -> (w34:T7)
  n116 = Obtain Notifier(name (unnamed)="Mixed Mode Statuses", notification data type=w97, error in (no error)=w62) -> (notifier out=w98:refnum<notifier>, error out=w13:errorcluster)  [unwired: 1 in, 1 out]
  n117 = call "MCL Data Transactions List.vi"() -> ("Transactions"=w3:string[])  [unwired: 11 in]
  n118 = call "MCL Volts Transactions List.vi"() -> ("Transactions"=w4:string[])  [unwired: 11 in]
  n119 = Initialize Array(w18, 18 ("dimension size"), 3 ("dimension size")) -> (w17:dbl[][])
  n120 = call "External Sensor Sensitivities DAO.vi"("Persistent DAO Actions"=Persistant_DAO_Actions."Get") -> ("Sensitivities Out"=w63:dbl[])  [unwired: 3 in, 7 out]
  n121 = Build Array(w34, w34) -> (w20:T7[])
  n122 = Obtain Queue(name (unnamed)="Parameter Changes", element data type=T35 {"Change State"=enum."Mixed Mode", "LBCB Number"=enum."LBCB1"} ("Parameter Changes"), error in (no error)=w13) -> (queue out=w106:refnum<queue>, error out=w84:errorcluster)  [unwired: 2 in, 1 out]
  n123 = while {
    shift-right: [w235] -> _
    shift-left: w20 -> [w234]
    tunnel: w63 -> [w260]
    shift-right: [w255] -> _
    shift-left: w98 -> [w256]
    tunnel: w97 -> [w254]
    tunnel: [w250] -> w89
    tunnel: w4 -> [w227]
    tunnel: w3 -> [w236]
    shift-right: [w214] -> _
    shift-left: w17 -> [w233]
    shift-right: [w226] -> _
    shift-left: _ -> [w225]
    tunnel: w3 -> [w224]
    stop <- w250 stop-if-true
    w219 = DAO_Actions."Set" ("DAO Actions")
    w216 = "/External/"
    # "Ramp time times a multiplier loosely aligned\nwith Nyquist's rule of thumb"
    # "Status Changes Loop"
    n124 = local read "L1 Cmd  Volts"() -> (w261:dbl[])
    n125 = local read "L2 Cmd  Volts"() -> (w240:dbl[])
    n126 = local read "Volts LVDT & LC"() -> (w239:dbl[][])
    n127 = local read "Servo Error"() -> (w238:dbl[][])
    n128 = local read "External Sensors"() -> (w218:dbl[])
    n129 = local read "Measurements"() -> (w241:T20[])
    n130 = local read "Rigid Connection"() -> (w223:bool)
    n131 = local read "Averaging"() -> (w229:bool)
    n132 = local read "Commands"() -> (w231:T2[])
    n133 = call "GetSamplingRate.vi"() -> ("Sampling"=w251:i32)
    n134 = local read "MixedModeStates"() -> (w246:T23)
    n135 = local write "Status Changes"(w251) -> ()
    n136 = Multiply(x=w218, y=w260) -> (x*y=w230:dbl[])
    n137 = case shown="\"Update Command\"" w246 {
      tunnel: [FALSE TRUE TRUE TRUE TRUE TRUE TRUE TRUE TRUE TRUE TRUE TRUE] -> w242
      frame "Init", Default {
      }
      frame "Start Iterative Stage" {
      }
      frame "Convergence Check" {
      }
      frame "Update Stiffness Jacobian" {
      }
      frame "Update Command" {
      }
      frame "Start Iterative Ramp" {
      }
      frame "Run Iterative Ramp" {
      }
      frame "Start Iterative Stabilize" {
      }
      frame "Iterative Stabilize" {
      }
      frame "Start Iterative Holding" {
      }
      frame "Iterative Holding" {
      }
      frame "Start Stabilize" {
      }
    }
    n138 = call "Average All.vi"("Rigid Connection"=w223, "Averaging"=w229, "Commands"=w231, "Measurements"=w241) -> ("Data"=w222:dbl[][])  [unwired: 7 in]
    n139 = call "Sample Averaging.vi"("Sample In"=w230, "Averaging"=w229) -> ("Sample Out"=w217:dbl[])  [unwired: 9 in]
    n140 = call "Pack Volts.vi"("Servo Error"=w238, "Volts LVDT & LC"=w239, "L2 Cmd  Volts"=w240, "L1 Cmd  Volts"=w261) -> ("Volts Data"=w228:dbl[][])  [unwired: 7 in]
    n141 = local read "Ramp Time"() -> (w259:u32)
    n142 = local read "Hold Period"() -> (w237:bool)
    n143 = call "Continuous Dataset.vi"("Group ID"=w216, "Data In"=w217, "DAO Actions"=w219) -> ()  [unwired: 7 in, 2 out]
    n144 = call "Volts Dataset.vi"("Group ID"=w216, "Data In"=w218, "DAO Actions"=w219) -> ()  [unwired: 7 in, 2 out]
    n145 = local read "Current Target"() -> (w245:T5[])
    n146 = local read "Iterative Target"() -> (w243:T5[])
    n147 = Multiply(x=w259, y=u32 2) -> (x*y=w257:u32)
    n148 = case shown="True" w237 {
      tunnel: w236 -> [_ w273]
      tunnel: [w264 w268] -> w214
      tunnel: w222 -> [_ w268]
      tunnel: [w265 w274] -> w235
      tunnel: w234 -> [w265 _]
      tunnel: w233 -> [w264 _]
      tunnel: w216 -> [_ w267]
      tunnel: w217 -> [_ w272]
      tunnel: [w263 w271] -> w226
      tunnel: w225 -> [w263 _]
      tunnel: w219 -> [_ w266]
      frame False {
      }
      frame True {
        n149 = call "MCL Filter Hold Data.vi"("Data"=w268) -> ("Mixed Mode Data"=w274:T7[])  [unwired: 10 in]
        n150 = call "Batchify All Data.vi"("Data"=w268) -> ("Data Out"=w270:dbl[][])  [unwired: 10 in]
        n151 = call "Hold Dataset.vi"("Group ID"=w267, "Data In"=w272, "DAO Actions"=w266) -> ("Data Out"=w271:dbl[])  [unwired: 7 in, 1 out]
        n152 = call "Batch Dataset Store.vi"("Data"=w270, "Dataset Source"=Dataset_Source."Hold", "Transactions"=w273) -> ()  [unwired: 8 in, 1 out]
      }
    }
    n153 = Wait Until Next ms Multiple(millisecond multiple=w257) -> ()  [unwired: 1 out]
    n154 = call "Batchify All Data.vi"("Data"=w222) -> ("Data Out"=w221:dbl[][])  [unwired: 10 in]
    n155 = Select(t=w243, s=w242, f=w245) -> (s? t:f=w244:T5[])
    n156 = local read "Convergence Status"() -> (w252:T22[])
    n157 = call "Batch Dataset Store.vi"("Data"=w221, "Dataset Source"=Dataset_Source."Continuous", "Transactions"=w224) -> ()  [unwired: 8 in, 1 out]
    n158 = call "Batch Dataset Store.vi"("Data"=w228, "Dataset Source"=Dataset_Source."Volts", "Transactions"=w227) -> ()  [unwired: 8 in, 1 out]
    n159 = call "MCL Filter Mixed Mode Data.vi"("Data"=w214) -> ("Mixed Mode Data"=w232:T12[])  [unwired: 10 in]
    n160 = Bundle By Name(cluster=w254, "LBCB Target"=w244, "MixedModeStates"=w246, "LBCB Convergence"=w252, "LBCB Measurements"=w232) -> (w253:T33)
    n161 = local read "App Running"() -> (w262:bool)
    n162 = local read "L1 Autobalance Out"() -> (w249:T8[])
    n163 = local read "L2 Autobalance Out"() -> (w248:T8[])
    n164 = Not(x=w262) -> (.not. x?=w250:bool)
    n165 = local write "Hold Data"(w235) -> ()
    n166 = Send Notification(notification=w253, notifier=w256) -> (notifier out=w255:refnum<notifier>)  [unwired: 1 in, 1 out]
    n167 = call "Autobalance Data DAO.vi"("L2 Autobalance In"=w248, "L1 Autobalance Iin"=w249, "DAO Actions"=DAO_Actions."Set") -> ()  [unwired: 1 in, 8 out]
  }
  n168 = Flush Queue(queue=w106, error in (no error)=w84) -> (queue out=w85:refnum<queue>, error out=w83:errorcluster)  [unwired: 1 out]
  n169 = flat-sequence {
    tunnel: [w292] -> w68
    tunnel: [w294] -> w67
    tunnel: [w293] -> w66
    tunnel: w13 -> [_]
    tunnel: [w287] -> w60
    frame #0 {
      n170 = global read "Global Cache.vi" "L2 Calibrations"() -> (w295:T46)
      n171 = Unbundle By Name(w295) -> ("Command Sensitivity"=w292:dbl[], "Servo Error Offset"=w287:dbl[], "LVDT Sensitivity"=w289:dbl[], "LVDT Offset"=w291:dbl[], "Load Cell Offsets"=w290:dbl[], "Load Cell Sensitivity"=w288:dbl[])
      n172 = Build Array (concatenate)(w291, w290) -> (w294:dbl[])
      n173 = Build Array (concatenate)(w289, w288) -> (w293:dbl[])
    }
  }
  n174 = call "Init Mixed Mode Command.vi"("error in (no error)"=w13) -> ("error out"=w15:errorcluster, "Command Data"=w80:T5)  [unwired: 1 out]
  n175 = Initialize Array(0.0 ("Numeric"), 6 ("dimension size")) -> (w23:dbl[])
  n176 = Bundle By Name(cluster=T7 {"Displacements"=[], "Forces"=[], "Displacement \nCommands"=[]} ("element"), "Displacements"=w23, "Forces"=w23, "Displacement \nCommands"=w23) -> (w25:T7)
  n177 = Bundle By Name(cluster=w57, "Command"=Mixed_Mode_Command_Action."No Op", "Ramp Times"=cluster{"Initial":T31, "Iterative":T31} {"Initial"={"Ramp"=0.0, "Stab"=0.0, "Hold"=0.0}, "Iterative"={"Ramp"=0.0, "Stab"=0.0, "Hold"=0.0}}, "LBCB1"=w80, "LBCB2"=w80) -> (w79:T34)
  n178 = Obtain Queue(name (unnamed)="Mixed Mode Commands", element data type=w57, error in (no error)=w13) -> (queue out=w105:refnum<queue>, error out=w102:errorcluster)  [unwired: 2 in, 1 out]
  n179 = Bundle By Name(cluster=T27 {"Act Disp"=[], "Act Forces"=[], "Cart Disp"=[], "Cart Forces"=[]} ("Measurements Out"), "Act Disp"=w23, "Act Forces"=w23) -> (w24:T27)
  n180 = Flush Queue(queue=w105, error in (no error)=w102) -> (queue out=w56:refnum<queue>, error out=w10:errorcluster)  [unwired: 1 out]
  n181 = while {
    shift-right: [w307] -> _
    shift-left: w85 -> [w310]
    shift-right: [w299] -> _
    shift-left: w83 -> [w309]
    tunnel: [w303] -> w90
    tunnel: w59 -> [w302]
    tunnel: w39 -> [w301]
    tunnel: w57 -> [w298]
    shift-right: [w296] -> _
    shift-left: w56 -> [w297]
    stop <- w303 stop-if-true
    # "Parameter Changes Loop"
    n182 = Dequeue Element(queue=w310, timeout in ms (-1)=2000, error in (no error)=w309) -> (queue out=w307:refnum<queue>, element=w306:T35, timed out?=w308:bool, error out=w300:errorcluster)
    n183 = case shown="False" w308 {
      tunnel: w306 -> [w320 _]
      tunnel: w302 -> [w317 _]
      tunnel: w301 -> [w316 _]
      tunnel: w300 -> [w315 w504]
      tunnel: [w314 w504] -> w299
      tunnel: w298 -> [w313 _]
      tunnel: w297 -> [w312 w505]
      tunnel: [w311 w505] -> w296
      frame False {
        n184 = Unbundle By Name(w320) -> ("Change State"=w319:T36, "LBCB Number"=w318:T28)
        n185 = case shown="\"Reset Auto-Balance\"" w319 {
          tunnel: w318 -> [_ _ _ _ _ _ w442 _ w453 w464 w497 _]
          tunnel: w317 -> [_ _ _ _ w420 _ _ _ _ _ _ _]
          tunnel: w316 -> [_ _ _ _ _ _ _ _ _ w465 _ _]
          tunnel: w315 -> [w335 w358 w364 w368 w399 w423 w445 w449 w452 w462 w496 w502]
          tunnel: [w335 w358 w364 w368 w399 w423 w445 w449 w452 w461 w496 w502] -> w314
          tunnel: w313 -> [_ _ _ _ _ _ _ _ _ w460 _ _]
          tunnel: w312 -> [w334 w357 w363 w367 w398 w422 w444 w448 w451 w459 w495 w501]
          tunnel: [w334 w357 w363 w367 w398 w422 w444 w448 w451 w458 w495 w501] -> w311
          frame "Mixed Mode" {
            w325 = LBCB_Number."LBCB2" ("LBCB Number")
            w326 = LBCB_Number."LBCB1" ("LBCB Number")
            w327 = Persistant_DAO_Actions."Get" ("LBCB Settings Actions")
            n186 = call "Mixed Mode Force Error Range DAO.vi"("Force Error Range Actions"=w327, "LBCB Number"=w326) -> ("Force Error Range Out"=w344:T39)  [unwired: 3 in, 10 out]
            n187 = call "Mixed Mode Jacobian Gain DAO.vi"("Jacobian Gain Actions"=w327, "LBCB Number"=w326) -> ("Jacobian Gain Out"=w343:T39)  [unwired: 3 in, 10 out]
            n188 = call "Mixed Mode Max Increment DAO.vi"("Max Increment Actions"=w327, "LBCB Number"=w326) -> ("Max Increment Out"=w342:T39)  [unwired: 3 in, 10 out]
            n189 = call "Cartesian Point 2 Array.vi"("Cart Disp"=w342) -> ("Array"=w339:dbl[])  [unwired: 2 out]
            n190 = call "Cartesian Point 2 Array.vi"("Cart Disp"=w343) -> ("Array"=w340:dbl[])  [unwired: 2 out]
            n191 = call "Cartesian Point 2 Array.vi"("Cart Disp"=w344) -> ("Array"=w341:dbl[])  [unwired: 2 out]
            n192 = call "Mixed Mode Max Increment DAO.vi"("Max Increment Actions"=w327, "LBCB Number"=w325) -> ("Max Increment Out"=w336:T39)  [unwired: 3 in, 10 out]
            n193 = call "Mixed Mode Force Error Range DAO.vi"("Force Error Range Actions"=w327, "LBCB Number"=w325) -> ("Force Error Range Out"=w338:T39)  [unwired: 3 in, 10 out]
            n194 = call "Mixed Mode Jacobian Gain DAO.vi"("Jacobian Gain Actions"=w327, "LBCB Number"=w325) -> ("Jacobian Gain Out"=w337:T39)  [unwired: 3 in, 10 out]
            n195 = call "Cartesian Point 2 Array.vi"("Cart Disp"=w338) -> ("Array"=w332:dbl[])  [unwired: 1 in, 1 out]
            n196 = call "Cartesian Point 2 Array.vi"("Cart Disp"=w337) -> ("Array"=w330:dbl[])  [unwired: 1 in, 1 out]
            n197 = call "Cartesian Point 2 Array.vi"("Cart Disp"=w336) -> ("Array"=w328:dbl[])  [unwired: 1 in, 1 out]
            n198 = call "Force Control Parameters DAO.vi"("DAO Actions"=w327) -> ("Force Control Parameters Out"=w324:T48)  [unwired: 8 in, 2 out]
            n199 = call "Mixed Mode Force Group Priorities DAO.vi"("Force Error Range Actions"=w327, "LBCB Number"=w326) -> ("Force Group Priorities Out"=w323:T49)  [unwired: 11 in, 2 out]
            n200 = call "Mixed Mode Force Group Priorities DAO.vi"("Force Error Range Actions"=w327, "LBCB Number"=w325) -> ("Force Group Priorities Out"=w322:T49)  [unwired: 11 in, 2 out]
            n201 = Build Array(w323, w322) -> (w321:T49[])
            n202 = local write item#-1(w321) -> ()
            n203 = Build Array(w341, w332) -> (w333:dbl[][])
            n204 = Build Array(w340, w330) -> (w331:dbl[][])
            n205 = Build Array(w339, w328) -> (w329:dbl[][])
            n206 = local write "Force Error Range"(w333) -> ()
            n207 = local write "Max Increment"(w329) -> ()
            n208 = local write "Jacobian Gain"(w331) -> ()
            n209 = local write item#-1(w324) -> ()
          }
          frame "Stiffness Jacobian" {
            w353 = cluster{T21} {[[1000000.0, 0.0, 0.0, 0.0, 0.0, 0.0], [0.0, 1000000.0, 0.0, 0.0, 0.0, 0.0], [0.0, 0.0, 1000000.0, 0.0, 0.0, 0.0], [0.0, 0.0, 0.0, 1000000.0, 0.0, 0.0], [0.0, 0.0, 0.0, 0.0, 1000000.0, 0.0], [0.0, 0.0, 0.0, 0.0, 0.0, 1000000.0]]} ("Cluster")
            w346 = LBCB_Number."LBCB1" ("LBCB Number")
            w345 = LBCB_Number."LBCB2" ("LBCB Number")
            w347 = Persistant_DAO_Actions."Get" ("Actions")
            n210 = call "Stiffness Limits DAO.vi"("Actions"=w347, "ID"=w345) -> ("Stiffness Limit Out"=w350:T42)  [unwired: 11 in, 2 out]
            n211 = call "Stiffness Limits DAO.vi"("Actions"=w347, "ID"=w346) -> ("Stiffness Limit Out"=w352:T42)  [unwired: 11 in, 2 out]
            n212 = call "Stiffness Jacobian DAO.vi"("LBCB Number"=w346, "Actions"=w347) -> ("Stiffness Jacobian Out"=w360:T21)  [unwired: 3 in, 6 out]
            n213 = call "Stiffness Jacobian DAO.vi"("LBCB Number"=w345, "Actions"=w347) -> ("Stiffness Jacobian Out"=w359:T21)  [unwired: 3 in, 6 out]
            n214 = call "Actuator Matrix 2 2D Array.vi"("Matrix In"=w350) -> ("Matrix Out"=w349:T19)  [unwired: 10 out]
            n215 = call "Actuator Matrix 2 2D Array.vi"("Matrix In"=w352) -> ("Matrix Out"=w351:T19)  [unwired: 10 out]
            n216 = call "Calculated Stiffness Jacobian.vi"("Stiffness Jacobian In"=w360, "LBCB Number"=w346, "Actions"=w347) -> ()  [unwired: 1 in, 8 out]
            n217 = call "Calculated Stiffness Jacobian.vi"("Stiffness Jacobian In"=w359, "LBCB Number"=w345, "Actions"=w347) -> ()  [unwired: 1 in, 8 out]
            n218 = Build Array(w351, w349) -> (w348:dbl[][][])
            n219 = local write "Stiffness Limits"(w348) -> ()
            n220 = Bundle(cluster=w353, w359) -> (w354:cluster{T21})
            n221 = Bundle(cluster=w353, w360) -> (w356:cluster{T21})
            n222 = Build Array(w356, w354) -> (w355:cluster{T21}[])
            n223 = local write "Stiffness Jacobian"(w355) -> ()
          }
          frame "Position" {
            n224 = call "Number Of LBCBs DAO.vi"("Actions"=Persistant_DAO_Actions."Get") -> ("Rigid Connection Out"=w361:bool)  [unwired: 4 in, 6 out]
            n225 = local write "Rigid Connection"(w361) -> ()
          }
          frame "Control Loop" {
            w370 = LBCB_Number."LBCB2" ("LBCB Number")
            w371 = LBCB_Number."LBCB1" ("LBCB Number")
            w369 = Persistant_DAO_Actions."Get" ("I Gain Actions")
            n226 = call "I Gain DAO.vi"("I Gain Actions"=w369, "LBCB Number"=w371) -> ("I Gain"=w380:T41)  [unwired: 3 in, 10 out]
            n227 = call "P Gain DAO.vi"("P Gain Actions"=w369, "LBCB Number"=w371) -> ("P Gain"=w379:T41)  [unwired: 3 in, 10 out]
            n228 = call "PID Controls DAO.vi"("Actions"=w369) -> ("PID Control  Out"=w376:T24)  [unwired: 3 in, 7 out]
            n229 = call "I Gain DAO.vi"("I Gain Actions"=w369, "LBCB Number"=w370) -> ("I Gain"=w374:T41)  [unwired: 3 in, 10 out]
            n230 = call "P Gain DAO.vi"("P Gain Actions"=w369, "LBCB Number"=w370) -> ("P Gain"=w375:T41)  [unwired: 3 in, 10 out]
            n231 = call "PID Controls DAO.vi"("Actions"=w369) -> ("PID Control  Out"=w365:T24)  [unwired: 3 in, 7 out]
            n232 = call "Actuator Point 2 Array.vi"("Actuator Point"=w380) -> ("Array"=w378:dbl[])
            n233 = call "Actuator Point 2 Array.vi"("Actuator Point"=w379) -> ("Array"=w377:dbl[])
            n234 = call "Actuator Point 2 Array.vi"("Actuator Point"=w374) -> ("Array"=w373:dbl[])
            n235 = call "Actuator Point 2 Array.vi"("Actuator Point"=w375) -> ("Array"=w372:dbl[])
            n236 = local write item#-1(w373) -> ()
            n237 = local write item#-1(w372) -> ()
            n238 = local write item#-1(w378) -> ()
            n239 = local write item#-1(w377) -> ()
            n240 = Build Array(w376, w365) -> (w366:T24[])
            n241 = local write "PID Control"(w366) -> ()
          }
          frame "Limits" {
            w390 = T2 {"Act Cmd"=[], "Cart Cmd"=[]} ("Data")
            w381 = LBCB_Number."LBCB2" ("ID")
            w383 = LBCB_Number."LBCB1" ("ID")
            w382 = Persistant_DAO_Actions."Get" ("Actuator Force Limit Actions")
            n242 = call "Command Voltage Limit DAO.vi"("Actuator Stroke Limit Actions"=w382, "ID"=w383) -> ("Command Voltage Limit Out"=w415:T40)  [unwired: 3 in, 10 out]
            n243 = call "Cartesian Increment Limits DAO.vi"("Actions"=w382, "LBCB Number"=w383) -> ("Inc Limits Out"=w392:T39)  [unwired: 11 in, 2 out]
            n244 = call "Actuator Force Limit DAO.vi"("Actuator Force Limit Actions"=w382, "ID"=w383) -> ("Actuator Force Limits Out"=w419:T40)  [unwired: 3 in, 10 out]
            n245 = call "Actuator Stroke Limit DAO.vi"("Actuator Stroke Limit Actions"=w382, "ID"=w383) -> ("Actuator Stroke Limits Out"=w418:T40)  [unwired: 3 in, 10 out]
            n246 = call "Cartesian Displacement Limit DAO.vi"("Cartesian Displacement Limit Actions"=w382, "ID"=w383) -> ("Cartesian Displacement Out"=w417:T42)  [unwired: 3 in, 10 out]
            n247 = call "Cartesian Force Limit DAO.vi"("Cartesian Force Limit Actions"=w382, "ID"=w383) -> ("Cartesian Force Limit Out"=w416:T42)  [unwired: 3 in, 10 out]
            n248 = call "Actuator Increment Limits DAO.vi"("Actions"=w382, "LBCB Number"=w383) -> ("Inc Limits Out"=w395:T41)  [unwired: 11 in, 2 out]
            n249 = call "Cartesian Point 2 Array.vi"("Cart Disp"=w392) -> ("Array"=w388:dbl[])  [unwired: 2 in]
            n250 = call "Cartesian Point 2 Array.vi"("Cart Disp"=w395) -> ("Array"=w389:dbl[])  [unwired: 2 in]
            n251 = call "Actuator Matrix 2 2D Array.vi"("Matrix In"=w415) -> ("Matrix Out"=w410:T19)  [unwired: 10 out]
            n252 = call "Cartesian Matrix 2 2D Array.vi"("Matrix In"=w417) -> ("Matrix Out"=w412:T19)  [unwired: 10 out]
            n253 = call "Actuator Matrix 2 2D Array.vi"("Matrix In"=w419) -> ("Matrix Out"=w414:T19)  [unwired: 10 out]
            n254 = call "Actuator Matrix 2 2D Array.vi"("Matrix In"=w418) -> ("Matrix Out"=w413:T19)  [unwired: 10 out]
            n255 = call "Cartesian Matrix 2 2D Array.vi"("Matrix In"=w416) -> ("Matrix Out"=w411:T19)  [unwired: 10 out]
            n256 = Bundle By Name(cluster=w420, "Actuator Force Limits"=w414, "Actuator Stroke Limits"=w413, "Cartesian Disp Limit"=w412, "Cartesian Force Limit"=w411, "Command Voltage Limit"=w410) -> (w421:T18)
            n257 = Bundle By Name(cluster=w390, "Act Cmd"=w389, "Cart Cmd"=w388) -> (w384:T2)
            n258 = call "Cartesian Increment Limits DAO.vi"("Actions"=w382, "LBCB Number"=w381) -> ("Inc Limits Out"=w391:T39)  [unwired: 11 in, 2 out]
            n259 = call "Actuator Increment Limits DAO.vi"("Actions"=w382, "LBCB Number"=w381) -> ("Inc Limits Out"=w394:T41)  [unwired: 11 in, 2 out]
            n260 = call "Command Voltage Limit DAO.vi"("Actuator Stroke Limit Actions"=w382, "ID"=w381) -> ("Command Voltage Limit Out"=w405:T40)  [unwired: 3 in, 10 out]
            n261 = call "Actuator Force Limit DAO.vi"("Actuator Force Limit Actions"=w382, "ID"=w381) -> ("Actuator Force Limits Out"=w409:T40)  [unwired: 3 in, 10 out]
            n262 = call "Actuator Stroke Limit DAO.vi"("Actuator Stroke Limit Actions"=w382, "ID"=w381) -> ("Actuator Stroke Limits Out"=w408:T40)  [unwired: 3 in, 10 out]
            n263 = call "Cartesian Displacement Limit DAO.vi"("Cartesian Displacement Limit Actions"=w382, "ID"=w381) -> ("Cartesian Displacement Out"=w407:T42)  [unwired: 3 in, 10 out]
            n264 = call "Cartesian Force Limit DAO.vi"("Cartesian Force Limit Actions"=w382, "ID"=w381) -> ("Cartesian Force Limit Out"=w406:T42)  [unwired: 3 in, 10 out]
            n265 = call "Cartesian Matrix 2 2D Array.vi"("Matrix In"=w406) -> ("Matrix Out"=w401:T19)  [unwired: 10 out]
            n266 = call "Cartesian Matrix 2 2D Array.vi"("Matrix In"=w407) -> ("Matrix Out"=w402:T19)  [unwired: 10 out]
            n267 = call "Cartesian Point 2 Array.vi"("Cart Disp"=w391) -> ("Array"=w386:dbl[])  [unwired: 2 in]
            n268 = call "Actuator Matrix 2 2D Array.vi"("Matrix In"=w405) -> ("Matrix Out"=w400:T19)  [unwired: 10 out]
            n269 = call "Actuator Matrix 2 2D Array.vi"("Matrix In"=w409) -> ("Matrix Out"=w404:T19)  [unwired: 10 out]
            n270 = call "Actuator Matrix 2 2D Array.vi"("Matrix In"=w408) -> ("Matrix Out"=w403:T19)  [unwired: 10 out]
            n271 = call "Cartesian Point 2 Array.vi"("Cart Disp"=w394) -> ("Array"=w387:dbl[])  [unwired: 2 in]
            n272 = Bundle By Name(cluster=w390, "Act Cmd"=w387, "Cart Cmd"=w386) -> (w385:T2)
            n273 = Bundle By Name(cluster=w420, "Actuator Force Limits"=w404, "Actuator Stroke Limits"=w403, "Cartesian Disp Limit"=w402, "Cartesian Force Limit"=w401, "Command Voltage Limit"=w400) -> (w396:T18)
            n274 = Build Array(w384, w385) -> (w393:T2[])
            n275 = Build Array(w421, w396) -> (w397:T18[])
            n276 = local write "Increment Limits"(w393) -> ()
            n277 = local write "Limits"(w397) -> ()
          }
          frame "Application" {
            w424 = 1000.0 ("x")
            n278 = call "App Parameters DAO.vi"("Actions"=Persistant_DAO_Actions."Get") -> ("Application Timing and Logging Out"=w430:T43)  [unwired: 3 in, 7 out]
            n279 = Unbundle By Name(w430) -> ("Ramp Time.Interval"=w429:dbl, "Logging Directory"=w427:path, "Volt Logging Loop.Interval"=w426:dbl)
            n280 = Multiply(x=w424, y=w426) -> (x*y=w425:dbl)
            n281 = Multiply(x=w424, y=w429) -> (x*y=w428:dbl)
            n282 = local write "Volt Logger Time"(w425) -> ()
            n283 = local write "Logging Directory"(w427) -> ()
            n284 = local write "Ramp Time"(w428) -> ()
          }
          frame "Reset Auto-Balance" {
            w436 = Persistant_DAO_Actions."Get" ("Auto Balance Increment Actions")
            n285 = case shown="\"LBCB2\"" w442 {
              tunnel: Control_Loop_State."Reset Autobalancing" ("L1 Ctrl Loop State") -> [w446 w447]
              frame "LBCB1", Default {
                n286 = local write "L1 Ctrl Loop State"(w446) -> ()
              }
              frame "LBCB2" {
                n287 = local write "L2 Ctrl Loop State"(w447) -> ()
              }
            }
            n288 = call "Autobalance Control DAO.vi"("Persistent DAO Actions"=Persistant_DAO_Actions."Get") -> ("Autobalance Control Out"=w440:T6)  [unwired: 8 in, 2 out]
            n289 = local write "AB Parameters"(w440) -> ()
            n290 = call "Auto Balance Error Tolerance DAO.vi"("Auto Balance Increment Actions"=w436, "LBCB Number"=LBCB_Number."LBCB1") -> ("Auto Balance Error Out"=w432:T41)  [unwired: 3 in, 10 out]
            n291 = call "Auto Balance Error Tolerance DAO.vi"("Auto Balance Increment Actions"=w436, "LBCB Number"=LBCB_Number."LBCB2") -> ("Auto Balance Error Out"=w433:T41)  [unwired: 3 in, 10 out]
            n292 = call "Actuator Point 2 Array.vi"("Actuator Point"=w433) -> ("Array"=w434:dbl[])
            n293 = call "Actuator Point 2 Array.vi"("Actuator Point"=w432) -> ("Array"=w438:dbl[])
            n294 = Build Array(w438, w434) -> (w439:dbl[][])
            n295 = local write "Auto Balance Error Tolerance"(w439) -> ()
          }
          frame "Stop Application" {
            n296 = local write "App Running"(FALSE ("App Running")) -> ()
          }
          frame "Set Command" {
            n297 = case shown="\"LBCB1\"" w453 {
              tunnel: Control_Loop_State."Set Command" ("L1 Ctrl Loop State") -> [w455 w456]
              frame "LBCB1" {
                n298 = local write "L1 Ctrl Loop State"(w455) -> ()
              }
              frame "LBCB2" {
                n299 = local write "L2 Ctrl Loop State"(w456) -> ()
              }
            }
          }
          frame "Enable Control" {
            n300 = case shown="\"LBCB2\"" w464 {
              tunnel: Control_Loop_State."On" ("L1 Ctrl Loop State") -> [w493 w494]
              tunnel: [w493 w494] -> w457
              frame "LBCB1" {
                n301 = local write "L1 Ctrl Loop State"(w493) -> ()
              }
              frame "LBCB2" {
                n302 = local write "L2 Ctrl Loop State"(w494) -> ()
              }
            }
            n303 = case shown="\"2\"" w465 {
              tunnel: w464 -> [_ w475]
              tunnel: w457 -> [_ w474]
              tunnel: w462 -> [w467 w472]
              tunnel: [w467 w471] -> w461
              tunnel: w460 -> [_ w470]
              tunnel: w459 -> [w466 w469]
              tunnel: [w466 w468] -> w458
              frame "1", Default {
              }
              frame "2" {
                n304 = case shown="\"LBCB1\"" w475 {
                  tunnel: w474 -> [w488 w491]
                  tunnel: [w487 w490] -> w473
                  frame "LBCB1" {
                    n305 = local read "L2 Ctrl Loop State"() -> (w489:T13)
                    n306 = Equal?(x=w488, y=w489) -> (x = y?=w487:bool)
                  }
                  frame "LBCB2" {
                    n307 = local read "L1 Ctrl Loop State"() -> (w492:T13)
                    n308 = Equal?(x=w491, y=w492) -> (x = y?=w490:bool)
                  }
                }
                n309 = case shown="True" w473 {
                  tunnel: w472 -> [w477 w486]
                  tunnel: [w477 w485] -> w471
                  tunnel: w470 -> [_ w483]
                  tunnel: w469 -> [w476 w482]
                  tunnel: [w476 w481] -> w468
                  frame False {
                  }
                  frame True {
                    n310 = call "Persistant Ramp Time DAO.vi"("Ramp Time Actions"=Persistant_DAO_Actions."Get") -> ("Ramp Time Out"=w478:T50)  [unwired: 12 in, 2 out]
                    n311 = Bundle By Name(cluster=w483, "Command"=Mixed_Mode_Command_Action."Measure Initial Position", "Ramp Times"=w478) -> (w484:T34)
                    n312 = Enqueue Element(queue=w482, element=w484, error in (no error)=w486) -> (queue out=w481:refnum<queue>, error out=w485:errorcluster)  [unwired: 1 in, 1 out]
                  }
                }
              }
            }
          }
          frame "Disable Control" {
            n313 = case shown="\"LBCB1\"" w497 {
              tunnel: Control_Loop_State."Ready for Control" ("L1 Ctrl Loop State") -> [w499 w500]
              frame "LBCB1" {
                n314 = local write "L1 Ctrl Loop State"(w499) -> ()
              }
              frame "LBCB2" {
                n315 = local write "L2 Ctrl Loop State"(w500) -> ()
              }
            }
          }
          frame "Start DAQ" {
            n316 = local write "DAQ Enabled"(TRUE ("DAQ Enabled")) -> ()
          }
        }
      }
      frame True {
        n317 = local read "L1 Ctrl Loop State"() -> (w511:T13)
        n318 = local read "L2 Ctrl Loop State"() -> (w508:T13)
        n319 = call "App Status Globals.vi"("App Status Actions"=App_Status_Actions."Get Status") -> ("App Status Out"=w515:T52)  [unwired: 5 in, 9 out]
        n320 = call "Control Loop State 2 Flags.vi"("L1 Ctrl Loop State"=w511) -> ("Controlled"=w509:bool, "Autobalanced"=w510:bool)
        n321 = local read "DAQ Started"() -> (w512:bool)
        n322 = call "Control Loop State 2 Flags.vi"("L1 Ctrl Loop State"=w508) -> ("Controlled"=w507:bool, "Autobalanced"=w506:bool)
        n323 = Bundle By Name(cluster=w515, "Controlling L2"=w507, "Autobalance L2"=w506, "Data Acquisition"=w512, "Controlling L1"=w509, "Autobalance L1"=w510) -> (w513:T52)
        n324 = call "App Status Globals.vi"("App Status Actions"=App_Status_Actions."Set All", "App Status In"=w513) -> ()  [unwired: 4 in, 10 out]
      }
    }
    n325 = local read "App Running"() -> (w305:bool)
    n326 = Not(x=w305) -> (.not. x?=w303:bool)
  }
  n327 = Obtain Queue(element data type=Command_or_Stiffness_Updates."Command Update" ("Command || Stiffness Update"), error in (no error)=w15) -> (queue out=w9:refnum<queue>, error out=w14:errorcluster)  [unwired: 3 in, 1 out]
  n328 = Initialize Array(0.0, 2 ("dimension size"), 6 ("dimension size")) -> (w28:dbl[][])
  n329 = Obtain Queue(name (unnamed)="Mixed Mode State", element data type=w104, error in (no error)=w14) -> (queue out=w94:refnum<queue>, error out=w101:errorcluster)  [unwired: 2 in, 1 out]
  n330 = Initialize Array(T14 {"Act Disp"={"X1"=TRUE, "X2"=TRUE, "Y1"=TRUE, "Z1"=TRUE, "Z2"=TRUE, "Z3"=TRUE}, "Act Force"={"X1"=TRUE, "X2"=TRUE, "Y1"=TRUE, "Z1"=TRUE, "Z2"=TRUE, "Z3"=TRUE}, "Act Incr"={"X1"=TRUE, "X2"=TRUE, "Y1"=TRUE, "Z1"=TRUE, "Z2"=TRUE, "Z3"=TRUE}, "Cart Disp"={"Dx"=TRUE, "Dy"=TRUE, "Dz"=TRUE, "Rx"=TRUE, "Ry"=TRUE, "Rz"=TRUE}, "Cart Force"={"Fx"=TRUE, "Fy"=TRUE, "Fz"=TRUE, "Mx"=TRUE, "My"=TRUE, "Mz"=TRUE}, "Cart Incr"={"Dx"=FALSE, "Dy"=FALSE, "Dz"=FALSE, "Rx"=FALSE, "Ry"=FALSE, "Rz"=FALSE}} ("Within Limits"), w38) -> (w41:T14[])
  n331 = Initialize Array(w25, w38) -> (w42:T7[])
  n332 = Initialize Array(w24, w38) -> (w43:T55)
  n333 = Build Array(LBCB_Number."LBCB1" ("LBCB Selected"), LBCB_Number."LBCB2" ("LBCB Selected")) -> (w52:T28[])
  n334 = while {
    shift-right: [w557] -> _
    shift-left: w104 -> [w550]
    shift-right: [w596] -> _
    shift-left: _ -> [w591]
    shift-right: [w594] -> _
    shift-left: u32 0 ("New Start Time") -> [w592]
    shift-right: [w590] -> _
    shift-left: w94 -> [w555]
    shift-right: [w585] -> _
    shift-left: w101 -> [w521]
    shift-right: [w551] -> _
    shift-left: w104 -> [w588]
    shift-right: [w586] -> _
    shift-left: w56 -> [w587]
    shift-right: [w582] -> _
    shift-left: w79 -> [w584]
    tunnel: [w579] -> w88
    tunnel: w39 -> [w578]
    shift-right: [w577] -> _
    shift-left: w43 -> [w545]
    shift-right: [w576] -> _
    shift-left: w37 -> [w543]
    shift-right: [w575] -> _
    shift-left: w42 -> [w572]
    tunnel: w52 -> [w542]
    shift-right: [w560] -> _
    shift-left: _ -> [w571]
    shift-right: [w561] -> _
    shift-left: _ -> [w570]
    shift-right: [w562] -> _
    shift-left: _ -> [w569]
    shift-right: [w558] -> _
    shift-left: w41 -> [w559]
    shift-right: [w549] -> _
    shift-left: w37 -> [w548]
    shift-right: [w541] -> _
    shift-left: _ -> [w540]
    shift-right: [w539] -> _
    shift-left: FALSE -> [w538]
    shift-right: [w525] -> _
    shift-left: w28 -> [w531]
    shift-right: [w524] -> _
    shift-left: w28 -> [w528]
    shift-right: [w522] -> _
    shift-left: w9 -> [w523]
    stop <- w579 stop-if-true
    # "Current Actuator\nPosition"
    # "Necessary because of \nthe PID loops"
    # "Make sure that overrides\nare broadcast and recorded"
    # "Needed for Convergence Check"
    # "Previous Hold Data"
    n335 = local read "Rigid Connection"() -> (w536:bool)
    n336 = Unbundle By Name(w584) -> ("Command"=w583:T32)
    n337 = local read "L1 Ctrl Loop Out Actuator"() -> (w529:dbl[])
    n338 = local read "L2 Ctrl Loop Out Actuator"() -> (w530:dbl[])
    n339 = case shown="\"Measure Initial Position\"" w583 {
      tunnel: w550 -> [w1418 _ _ w1421 w1422 w1423]
      tunnel: [w1418 Mixed_Mode_States."Aborting" ("MixedModeStates") Mixed_Mode_States."Exit" ("MixedModeStates") w1421 w1422 w1423] -> w551
      frame "Start Command" {
      }
      frame "Stop" {
      }
      frame "Exit" {
      }
      frame "No Op" {
      }
      frame "Start Acquisition" {
      }
      frame "Measure Initial Position" {
      }
    }
    n340 = call "Current Position DAO.vi"("Rigid Connection"=w536, "Actions"=DAO_Actions."Get") -> ("LBCB 2 Commands Out"=w532:dbl[], "LBCB 1 Commands Out"=w533:dbl[])  [unwired: 8 in]
    n341 = call "Ramp Timer.vi"("Previous Ramp Time"=w592) -> ("New Start Time"=w593:u32, "Current Ramp Time"=w595:u64)
    n342 = Replace Array Subset(array=w531, new element #1=w533, index (row) #1=0 ("index"), new element #2=w532, index (row) #2=1 ("index")) -> (w525:dbl[][])  [unwired: 2 in]
    n343 = Replace Array Subset(array=w528, new element #1=w529, index (row) #1=0 ("index (row)"), new element #2=w530, index (row) #2=1 ("index (row)")) -> (w524:dbl[][])  [unwired: 2 in]
    n344 = local read "Ramp Time"() -> (w573:u32)
    n345 = case shown="\"Update Stiffness Jacobian\"" w551 {
      tunnel: [Mixed_Mode_States."Wait For DAQ" ("f") w636 Mixed_Mode_States."Done" ("f") w687 Mixed_Mode_States."Initial Position" ("MixedModeStates") w706 w757 w803 w832 w884 Mixed_Mode_States."Convergence Check" ("MixedModeStates") Mixed_Mode_States."Start Iterative Ramp" ("MixedModeStates") Mixed_Mode_States."Run Iterative Ramp" ("MixedModeStates") w1026 Mixed_Mode_States."Iterative Stabilize" ("MixedModeStates") w1063 Mixed_Mode_States."Iterative Holding" ("MixedModeStates") w1095 Mixed_Mode_States."Stabilize" ("MixedModeStates") w1127 Mixed_Mode_States."Holding" ("MixedModeStates") w1159 Mixed_Mode_States."Idle" ("f") Mixed_Mode_States."Exit" ("f") Mixed_Mode_States."Idle" ("f")] -> w556
      tunnel: [T31 {"Ramp"=0.0, "Stab"=0.0, "Hold"=0.0} ("Initial") w638 w670 w691 w699 w727 w761 w820 w851 w890 w929 w976 w1015 w1037 w1057 w1072 w1090 w1109 w1121 w1136 w1154 w1173 w1187 w1195 w1208] -> w596
      tunnel: w595 -> [_ _ _ _ _ w724 _ w806 _ _ _ _ _ w1039 _ w1074 _ w1106 _ w1138 _ w1170 _ _ _]
      tunnel: [w613 w637 w669 w690 w702 w728 w766 w821 w849 w889 w928 w975 w1016 w1038 w1058 w1080 w1089 w1112 w1122 w1144 w1153 w1176 w1186 w1197 w1206] -> w594
      tunnel: w593 -> [_ _ _ _ w702 _ w766 _ _ _ _ _ w1016 _ w1058 _ w1089 _ w1122 _ w1153 _ _ _ _]
      tunnel: w592 -> [w613 w637 w669 w690 _ w728 _ w821 w849 w889 w928 w975 _ w1038 _ w1080 _ w1112 _ w1144 _ w1176 w1186 w1197 w1206]
      tunnel: w591 -> [_ w638 w670 w691 _ w727 _ w820 w851 w890 w929 w976 _ w1037 _ w1072 w1090 w1109 _ w1136 w1154 w1173 w1187 w1195 w1208]
      tunnel: w583 -> [_ w625 _ w688 _ _ _ _ _ _ _ _ _ _ _ _ _ _ _ _ _ _ _ _ _]
      tunnel: w588 -> [_ _ _ _ _ _ _ _ _ _ _ _ _ _ _ _ _ _ _ _ _ _ _ _ _]
      tunnel: w587 -> [w610 w634 w667 w683 w701 w720 w765 w815 w848 w888 w926 w973 w1010 w1034 w1056 w1069 w1087 w1101 w1120 w1133 w1152 w1165 w1184 w1193 w1205]
      tunnel: [w610 w633 w667 w682 w701 w719 w765 w814 w848 w888 w926 w973 w1010 w1033 w1056 w1068 w1087 w1100 w1120 w1132 w1152 w1164 w1184 w1193 w1205] -> w586
      tunnel: [w608 w632 w665 w681 w698 w717 w764 w812 w847 w887 w927 w972 w1009 w1031 w1055 w1066 w1088 w1098 w1119 w1130 w1151 w1162 w1185 w1194 w1204] -> w582
      tunnel: w584 -> [w609 w629 w666 w678 w700 w718 w762 w813 w847 w887 w927 w972 w1009 w1032 w1055 w1067 w1088 w1099 w1119 w1131 w1151 w1163 w1185 w1194 w1204]
      tunnel: [_ _ _ _ _ w712 _ w818 _ _ _ _ _ w1028 _ _ _ _ _ _ _ _ _ _ _] -> w574
      tunnel: w578 -> [_ _ w664 _ _ w714 _ w811 _ _ _ _ _ w1030 _ _ _ _ _ _ _ _ _ _ _]
      tunnel: [w601 w620 w663 w675 w694 w715 w755 w810 w842 w882 w921 w963 w1008 w1027 w1054 w1064 w1086 w1096 w1118 w1128 w1150 w1160 w1183 w1192 w1202] -> w547
      tunnel: w573 -> [_ w623 w659 w677 _ w716 _ w809 _ _ _ _ _ w1029 _ w1065 _ w1097 _ w1129 _ w1161 w1181 _ _]
      tunnel: w542 -> [_ _ _ _ _ _ _ _ w843 w873 _ w967 _ _ _ _ _ _ _ _ _ _ _ _ _]
      tunnel: w572 -> [_ _ _ _ _ _ _ _ _ _ w923 _ _ _ _ _ _ _ _ _ _ _ _ _ _]
      tunnel: w536 -> [_ _ w646 _ _ w708 _ w802 _ _ _ _ _ w1020 _ _ _ _ _ _ _ _ _ _ _]
      tunnel: [w600 w619 w658 w674 w696 w711 w754 w801 w839 w875 w917 w960 w1006 w1025 w1052 w1062 w1084 w1094 w1116 w1126 w1148 w1158 w1180 w1191 w1201] -> w541
      tunnel: w540 -> [w600 w619 w658 w674 w696 w711 w754 w801 _ w875 w917 w960 w1006 w1025 w1052 w1062 w1084 w1094 w1116 w1126 w1148 w1158 w1180 w1191 w1201]
      tunnel: [w599 w618 w657 w673 w695 w710 w753 w800 FALSE w874 w916 TRUE w1005 w1024 w1051 w1061 w1083 w1093 w1115 w1125 w1147 w1157 w1179 w1190 w1200] -> w539
      tunnel: w538 -> [w599 w618 w657 w673 w695 w710 w753 w800 _ w874 w916 _ w1005 w1024 w1051 w1061 w1083 w1093 w1115 w1125 w1147 w1157 w1179 w1190 w1200]
      tunnel: w524 -> [_ _ w649 _ _ w709 _ _ _ _ _ _ _ _ _ _ _ _ _ _ _ _ _ _ _]
      tunnel: w525 -> [_ _ _ _ _ _ w752 w799 _ _ _ w958 _ w1023 _ _ _ _ _ _ _ _ _ _ _]
      tunnel: w523 -> [w598 w617 w645 w672 w693 w707 w750 w798 w834 w872 w912 w957 w1004 w1022 w1050 w1060 w1082 w1092 w1114 w1124 w1146 w1156 w1178 w1189 w1199]
      tunnel: [w598 w617 w645 w672 w693 w707 w749 w798 w833 w872 w911 w957 w1003 w1022 w1050 w1060 w1082 w1092 w1114 w1124 w1146 w1156 w1178 w1189 w1199] -> w522
      tunnel: w521 -> [w597 w616 w643 w671 w692 w705 w744 w796 w828 w870 w910 w956 w1001 w1019 w1049 w1059 w1081 w1091 w1113 w1123 w1145 w1155 w1177 w1188 w1198]
      tunnel: [w597 w616 w642 w671 w692 w704 w744 w795 w828 w870 w910 w956 w1001 w1018 w1049 w1059 w1081 w1091 w1113 w1123 w1145 w1155 w1177 w1188 w1198] -> w519
      frame "Init" {
        n346 = call "Init Mixed Mode Command.vi"() -> ("Command Data"=w605:T5)  [unwired: 1 in, 2 out]
        n347 = Build Array(MM_Result_Actions."Nop" ("MM Result Actions")) -> (w601:T1[])
        n348 = call "Mixed Mode Commands DAO.vi"("Mixed Mode Commands\n Datastore Actions"=DAO_Actions."Init" ("Mixed Mode Commands\n Datastore Actions")) -> ()  [unwired: 3 in, 8 out]
        n349 = Bundle By Name(cluster=w609, "Command"=Mixed_Mode_Command_Action."No Op", "Ramp Times"=cluster{"Initial":T31, "Iterative":T31} {"Initial"={"Ramp"=0.0, "Stab"=0.0, "Hold"=0.0}, "Iterative"={"Ramp"=0.0, "Stab"=0.0, "Hold"=0.0}}, "LBCB1"=w605, "LBCB2"=w605) -> (w608:T34)
        n350 = call "Stiffness Jacobian DAO.vi"("LBCB Number"=LBCB_Number."LBCB1" ("LBCB Selected"), "Actions"=Persistant_DAO_Actions."Init" ("Stiffness Jacobian Datastore Actions")) -> ()  [unwired: 3 in, 7 out]
        n351 = call "Convergence Status DAO.vi"("Actions"=Persistant_DAO_Actions."Init") -> ()  [unwired: 3 in, 8 out]
      }
      frame "Idle" {
        w620 = T1[] [enum."Check Limits"] items=["Nop", "Set Command", "Check Limits", "Send Command", "Store Prev Reading", "Averaging On", "Averaging Off", "Hold On", "Hold Off", "PID Hold On", "PID Hold Off", "Clear Increment Faults", "Set Initial Position"]
        n352 = Equal?(x=w625, y=Mixed_Mode_Command_Action."Measure Initial Position") -> (x = y?=w622:bool)
        n353 = Dequeue Element(queue=w634, timeout in ms (-1)=w623) -> (queue out=w633:refnum<queue>, element=w630:T34, timed out?=w631:bool)  [unwired: 1 in, 1 out]
        n354 = Select(t=Mixed_Mode_States."Start Initial Position", s=w622, f=Mixed_Mode_States."Idle" ("MixedModeStates")) -> (s? t:f=w626:T23)
        n355 = Equal?(x=Mixed_Mode_Command_Action."Start Command", y=w625) -> (x = y?=w621:bool)
        n356 = Select(t=w629, s=w631, f=w630) -> (s? t:f=w632:T34)
        n357 = case shown="True" w621 {
          tunnel: [w639 Mixed_Mode_States."Start Initial Ramp" ("MixedModeStates")] -> w636
          tunnel: w626 -> [w639 _]
          frame False {
          }
          frame True {
            n358 = call "Ramp Time DAO.vi"("Actions"=DAO_Actions."Init") -> ()  [unwired: 8 in, 3 out]
          }
        }
      }
      frame "Aborting" {
        w663 = T1[] [enum."Averaging Off", enum."Hold Off", enum."PID Hold Off"] items=["Nop", "Set Command", "Check Limits", "Send Command", "Store Prev Reading", "Averaging On", "Averaging Off", "Hold On", "Hold Off", "PID Hold On", "PID Hold Off", "Clear Increment Faults", "Set Initial Position"]
        n359 = Wait Until Next ms Multiple(millisecond multiple=w659) -> ()  [unwired: 1 out]
        n360 = call "Cntrl Loop Actuator Out 2 MM Comand.vi"("Act Cmds In"=w649, "Number of\nLBCBs In"=w664, "error in (no error)"=w643) -> ("Cmd Out"=w648:T2[], "error out"=w642:errorcluster)  [unwired: 11 in]
        n361 = call "Rigid Connection Command Reverse Filter.vi"("Rigid Connection"=w646, "LBCB Commands In"=w648) -> ("LBCB Commands Out"=w647:T2[])  [unwired: 9 in]
        n362 = call "Initial Target.vi"("Initial Position"=w647) -> ("Initial Target"=w661:T5[])
        n363 = Index Array(array=w648, index #1=0 ("index"), index #2=1 ("index")) -> (element #1=w653:T2, element #2=w652:T2)
        n364 = Bundle By Name(cluster=w666, "Command"=Mixed_Mode_Command_Action."No Op") -> (w665:T34)
        n365 = Unbundle By Name(w652) -> ("Cart Cmd"=w650:dbl[])
        n366 = Unbundle By Name(w653) -> ("Cart Cmd"=w651:dbl[])
        n367 = call "Mixed Mode Commands DAO.vi"("Current Target In"=w661, "Mixed Mode Commands\n Datastore Actions"=DAO_Actions."Set" ("Mixed Mode Commands\n Datastore Actions")) -> ("Current Target"=w660:T5[])  [unwired: 7 in, 2 out]
        n368 = local write "Current Target"(w660) -> ()
        n369 = call "Current Position DAO.vi"("Rigid Connection"=w646, "LBCB 2 Commands In"=w650, "LBCB 1 Commands In"=w651, "Actions"=DAO_Actions."Set") -> ()  [unwired: 6 in, 2 out]
      }
      frame "Wait For DAQ" {
        n370 = Build Array(MM_Result_Actions."Nop" ("MM Result Actions")) -> (w675:T1[])
        n371 = Dequeue Element(queue=w683, timeout in ms (-1)=w677) -> (queue out=w682:refnum<queue>, element=w679:T34, timed out?=w680:bool)  [unwired: 1 in, 1 out]
        n372 = Select(t=w678, s=w680, f=w679) -> (s? t:f=w681:T34)
        n373 = Equal?(x=Mixed_Mode_Command_Action."Start Acquisition", y=w688) -> (x = y?=w684:bool)
        n374 = Select(t=Mixed_Mode_States."Idle" ("MixedModeStates"), s=w684, f=Mixed_Mode_States."Wait For DAQ" ("MixedModeStates")) -> (s? t:f=w687:T23)
      }
      frame "Start Initial Position" {
        w694 = T1[] [enum."Averaging On", enum."Hold On"] items=["Nop", "Set Command", "Check Limits", "Send Command", "Store Prev Reading", "Averaging On", "Averaging Off", "Hold On", "Hold Off", "PID Hold On", "PID Hold Off", "Clear Increment Faults", "Set Initial Position"]
        n375 = Unbundle By Name(w700) -> ("Ramp Times.Initial"=w699:T31)
        n376 = Bundle By Name(cluster=w700, "Command"=Mixed_Mode_Command_Action."No Op") -> (w698:T34)
      }
      frame "Initial Position" {
        w715 = T1[] [enum."Averaging On", enum."Hold On", enum."Set Initial Position", enum."Check Limits"] items=["Nop", "Set Command", "Check Limits", "Send Command", "Store Prev Reading", "Averaging On", "Averaging Off", "Hold On", "Hold Off", "PID Hold On", "PID Hold Off", "Clear Increment Faults", "Set Initial Position"]
        n377 = Unbundle By Name(w727) -> ("Hold"=w723:dbl)
        n378 = Divide(x=w724, y=u64 1000) -> (x/y=w726:dbl)
        n379 = Greater?(x=w726, y=w723) -> (0:w713:bool)
        n380 = Dequeue Element(queue=w720, timeout in ms (-1)=w716) -> (queue out=w719:refnum<queue>, element=w721:T34, timed out?=w722:bool)  [unwired: 1 in, 1 out]
        n381 = call "Cntrl Loop Actuator Out 2 MM Comand.vi"("Act Cmds In"=w709, "Number of\nLBCBs In"=w714, "error in (no error)"=w705) -> ("Cmd Out"=w712:T2[], "error out"=w704:errorcluster)  [unwired: 11 in]
        n382 = case shown="True" w713 {
          tunnel: w712 -> [_ w737]
          tunnel: w708 -> [_ w730]
          tunnel: [Mixed_Mode_States."Initial Position" ("f") Mixed_Mode_States."Done" ("MixedModeStates")] -> w706
          frame False {
          }
          frame True {
            w738 = DAO_Actions."Set" ("Mixed Mode Commands\n Datastore Actions")
            n383 = Index Array(array=w737, index #1=0 ("index"), index #2=1 ("index")) -> (element #1=w734:T2, element #2=w732:T2)
            n384 = call "Rigid Connection Command Reverse Filter.vi"("Rigid Connection"=w730, "LBCB Commands In"=w737) -> ("LBCB Commands Out"=w741:T2[])  [unwired: 9 in]
            n385 = call "Commands 2 Cart Commands.vi"("Cmd In"=w737) -> ("Cart Commands Out"=w742:dbl[][])  [unwired: 10 in]
            n386 = Unbundle By Name(w734) -> ("Cart Cmd"=w733:dbl[])
            n387 = Unbundle By Name(w732) -> ("Cart Cmd"=w731:dbl[])
            n388 = call "Initial Target.vi"("Initial Position"=w741) -> ("Initial Target"=w743:T5[])
            n389 = call "Start Position DAO.vi"("Displacements In"=w742, "DAO Actions"=w738) -> ()  [unwired: 8 in, 2 out]
            n390 = call "Current Position DAO.vi"("Rigid Connection"=w730, "LBCB 2 Commands In"=w731, "LBCB 1 Commands In"=w733, "Actions"=w738) -> ()  [unwired: 6 in, 2 out]
            n391 = call "Mixed Mode Commands DAO.vi"("Current Target In"=w743, "Mixed Mode Commands\n Datastore Actions"=w738) -> ("Current Target"=w740:T5[])  [unwired: 7 in, 2 out]
            n392 = local write "Current Target"(w740) -> ()
            n393 = local write "Target"(w740) -> ()
          }
        }
        n394 = Select(t=w718, s=w722, f=w721) -> (s? t:f=w717:T34)
      }
      frame "Start Initial Ramp" {
        w755 = T1[] [enum."Clear Increment Faults"] items=["Nop", "Set Command", "Check Limits", "Send Command", "Store Prev Reading", "Averaging On", "Averaging Off", "Hold On", "Hold Off", "PID Hold On", "PID Hold Off", "Clear Increment Faults", "Set Initial Position"]
        # "The idea is that the initial position is fed into the target DAO and maintained for\nall DOFs that are not being commanded for displacement"
        n395 = Unbundle By Name(w762) -> ("Ramp Times.Initial"=w761:T31, "LBCB1"=w760:T5, "LBCB2"=w758:T5)
        n396 = Build Array(w760, w758) -> (w756:T5[])
        n397 = for {
          tunnel: w756 -> [w779] mode=indexing
          tunnel: [w781] -> w759 mode=indexing
          tunnel: w752 -> [w778] mode=indexing
          tunnel: [w776] -> w745 mode=indexing
          n398 = Unbundle By Name(w779) -> ("Command Type"=w782:enum16{"<None>", "Displacement", "Force"}[], "Displacements"=w780:dbl[])
          n399 = for {
            tunnel: w782 -> [w787] mode=indexing
            tunnel: [w789] -> w781 mode=indexing
            tunnel: w778 -> [w784] mode=indexing
            shift-right: [w783] -> w777
            shift-left: w780 -> [w786]
            i -> [w785]
            n400 = case shown="\"Force\", Default" w787 {
              tunnel: w786 -> [w790 w794]
              tunnel: [w790 w791] -> w783
              tunnel: w785 -> [_ w793]
              tunnel: w784 -> [_ w792]
              frame "Displacement" {
              }
              frame "Force", Default {
                # "Add Current\nDisp for Force\nControl"
                n401 = Replace Array Subset(array=w794, new element=w792, index=w793) -> (w791:dbl[])
              }
            }
            n402 = Equal?(x=enum16{"<None>", "Displacement", "Force"}."Displacement", y=w787) -> (x = y?=w789:bool)
          }
          n403 = Bundle By Name(cluster=w779, "Displacements"=w777) -> (w776:T5)
        }
        n404 = Unbundle By Name(w761) -> ("Ramp"=w769:dbl)
        n405 = Equal To 0?(x=w769) -> (x = 0?=w768:bool)
        n406 = Or Array Elements(Boolean array=w759) -> (logical OR=w751:bool)
        n407 = case shown="True" w751 {
          tunnel: w750 -> [w771 w775]
          tunnel: [w771 w773] -> w749
          tunnel: [Mixed_Mode_States."Start Iterative Stage" ("MixedModeStates") Mixed_Mode_States."Run Initial Ramp" ("MixedModeStates")] -> w748
          frame False {
          }
          frame True {
            n408 = Enqueue Element(queue=w775, element=Command_or_Stiffness_Updates."Command Update") -> (queue out=w773:refnum<queue>)  [unwired: 2 in, 2 out]
          }
        }
        n409 = call "Mixed Mode Commands DAO.vi"("Current Target In"=w745, "Mixed Mode Commands\n Datastore Actions"=DAO_Actions."Set" ("Mixed Mode Commands\n Datastore Actions")) -> ("Current Target"=w746:T5[])  [unwired: 3 in, 6 out]
        n410 = local write "Current Target"(w746) -> ()
        n411 = Bundle By Name(cluster=w762, "Command"=Mixed_Mode_Command_Action."No Op") -> (w764:T34)
        n412 = Select(t=Mixed_Mode_States."Idle" ("MixedModeStates"), s=w768, f=w748) -> (s? t:f=w757:T23)
      }
      frame "Run Initial Ramp" {
        w810 = T1[] [enum."Set Command", enum."Check Limits", enum."Send Command"] items=["Nop", "Set Command", "Check Limits", "Send Command", "Store Prev Reading", "Averaging On", "Averaging Off", "Hold On", "Hold Off", "PID Hold On", "PID Hold Off", "Clear Increment Faults", "Set Initial Position"]
        n413 = call "Ramp Time DAO.vi"("Actions"=DAO_Actions."Get") -> ("Ramp Time Out"=w807:u64)  [unwired: 8 in, 2 out]
        n414 = Add(x=w807, y=w806) -> (x+y=w805:u64)
        n415 = call "Ramp Time Completions.vi"("Current Ramp Time"=w805, "Initial"=w820) -> ("Still in Ramp"=w804:bool, "Fraction\nCompleted"=w819:dbl)
        n416 = case shown="False" w804 {
          tunnel: w819 -> [w824 _]
          tunnel: [Mixed_Mode_States."Run Initial Ramp" ("MixedModeStates") Mixed_Mode_States."Start Iterative Stage" ("MixedModeStates")] -> w803
          tunnel: [w822 w826] -> w797
          frame True {
            n417 = call "Calculate Ramp Displacements.vi"("Ramp Time"=w824) -> ("Target"=w822:T5[])  [unwired: 2 in]
          }
          frame False {
            n418 = call "Mixed Mode Commands DAO.vi"("Mixed Mode Commands\n Datastore Actions"=DAO_Actions."Get" ("Mixed Mode Commands\n Datastore Actions")) -> ("Current Target"=w826:T5[])  [unwired: 3 in, 7 out]
          }
        }
        n419 = Dequeue Element(queue=w815, timeout in ms (-1)=w809) -> (queue out=w814:refnum<queue>, element=w817:T34, timed out?=w816:bool)  [unwired: 1 in, 1 out]
        n420 = Select(t=w813, s=w816, f=w817) -> (s? t:f=w812:T34)
        n421 = local write "Target"(w797) -> ()
        n422 = call "MM Command to Cntrl Loop Actuator In.vi"("Target"=w797, "Current Cartesian Position"=w799, "Number of\nLBCBs In"=w811, "error in (no error)"=w796, "Rigid Connection"=w802) -> ("Cmd Out"=w818:T2[], "error out"=w795:errorcluster)  [unwired: 6 in, 3 out]
      }
      frame "Start Iterative Stage" {
        w842 = T1[] [enum."Check Limits", enum."Store Prev Reading"] items=["Nop", "Set Command", "Check Limits", "Send Command", "Store Prev Reading", "Averaging On", "Averaging Off", "Hold On", "Hold Off", "PID Hold On", "PID Hold Off", "Clear Increment Faults", "Set Initial Position"]
        # "Store Force Parameters for \nthis cycle of force ramps"
        # "Initialize the Multi DOF State Machine"
        # "Transfer Current Displacement to the Force Target"
        n423 = Unbundle By Name(w847) -> ("LBCB1"=w846:T5, "LBCB2"=w844:T5)
        n424 = Build Array(w846, w844) -> (w845:T5[])
        n425 = for {
          tunnel: T22 {"IsConverged"=[], "Force Errors"=[], "Controlling DOF"=[]} ("Convergence Status Out") -> [w865]
          tunnel: w845 -> [w860] mode=indexing
          tunnel: [w858] -> w841 mode=indexing
          tunnel: w843 -> [w857] mode=indexing
          tunnel: [w856] -> w835 mode=indexing
          n426 = Unbundle By Name(w860) -> ("Command Type"=w866:enum16{"<None>", "Displacement", "Force"}[])
          n427 = for {
            tunnel: w866 -> [w867] mode=indexing
            tunnel: [w869] -> w856 mode=indexing
            n428 = Not Equal?(x=enum16{"<None>", "Displacement", "Force"}."Force", y=w867) -> (x != y?=w869:bool)
          }
          n429 = Initialize Array(0.0 ("element"), 6 ("dimension size")) -> (w861:dbl[])
          n430 = Bundle By Name(cluster=w865, "IsConverged"=w856, "Force Errors"=w861) -> (w864:T22)
          n431 = call "Convergence Status DAO.vi"("Convergence Status In"=w864, "LBCB Selected"=w857, "Actions"=Persistant_DAO_Actions."Set") -> ("Convergence Status Out"=w858:T22)  [unwired: 1 in, 7 out]
        }
        n432 = Or Array Elements(Boolean array=w835) -> (logical OR=w831:bool)
        n433 = local read item#-1() -> (w839)
        n434 = case shown="True" w831 {
          tunnel: w834 -> [w852 w855]
          tunnel: [w852 w853] -> w833
          frame False {
          }
          frame True {
            n435 = Enqueue Element(queue=w855, element=Command_or_Stiffness_Updates."Command Update") -> (queue out=w853:refnum<queue>)  [unwired: 2 in, 2 out]
          }
        }
        n436 = call "MM Multi DOF Status DAO.vi"("Actions"=DAO_Actions."Init") -> ("error out"=w837:errorcluster)  [unwired: 9 in, 1 out]
        n437 = call "MM Multi DOF State Machine.vi"("error in (no error)"=w837, "Force Control Parameters"=w839, "Convergence Status In"=w841) -> ("Convergence Status Out"=w840:T22[])  [unwired: 7 in, 1 out]
        n438 = local write "Convergence Status"(w840) -> ()
        n439 = Select(t=Mixed_Mode_States."Start Iterative Stabilize", s=w831, f=Mixed_Mode_States."Start Stabilize" ("MixedModeStates")) -> (s? t:f=w832:T23)
      }
      frame "Convergence Check" {
        w882 = T1[] [enum."Hold Off", enum."Averaging Off"] items=["Nop", "Set Command", "Check Limits", "Send Command", "Store Prev Reading", "Averaging On", "Averaging Off", "Hold On", "Hold Off", "PID Hold On", "PID Hold Off", "Clear Increment Faults", "Set Initial Position"]
        n440 = local read "Hold Data"() -> (w883:T7[])
        n441 = call "Mixed Mode Commands DAO.vi"("Mixed Mode Commands\n Datastore Actions"=DAO_Actions."Get" ("Mixed Mode Commands\n Datastore Actions")) -> ("Current Target"=w885:T5[])  [unwired: 3 in, 7 out]
        n442 = local read "Force Error Range"() -> (w881:dbl[][])
        n443 = for {
          tunnel: [w903] -> w877 mode=indexing
          tunnel: w881 -> [w905] mode=indexing
          tunnel: w885 -> [w908] mode=indexing
          tunnel: w883 -> [w907] mode=indexing
          tunnel: w873 -> [w902] mode=indexing
          n444 = Unbundle By Name(w907) -> ("Forces"=w906:dbl[])
          n445 = call "Convergence Status DAO.vi"("LBCB Selected"=w902, "Actions"=DAO_Actions."Get") -> ("Convergence Status Out"=w909:T22)  [unwired: 2 in, 7 out]
          n446 = call "Convergence Check.vi"("Forces Error \nTolerances"=w905, "Command Data"=w908, "Cart\nForces"=w906, "Mixed Mode Convergence Status In"=w909) -> ("Mixed Mode Convergence Status Out"=w903:T22)  [unwired: 2 in, 5 out]
        }
        n447 = local read item#-1() -> (w880)
        n448 = call "MM Multi DOF State Machine.vi"("Force Control Parameters"=w875, "Convergence Status In"=w877) -> ("Convergence Status Out"=w876:T22[])  [unwired: 8 in, 1 out]
        n449 = for {
          tunnel: w881 -> [w899] mode=indexing
          tunnel: w880 -> [w898]
          tunnel: w876 -> [w897] mode=indexing
          tunnel: w873 -> [w893] mode=indexing
          tunnel: [w896] -> w879 mode=indexing
          tunnel: [w895] -> w878 mode=indexing
          tunnel: w875 -> [w894]
          n450 = call "Pick A DOF.vi"("LBCB Number"=w893, "Force Control Parameters"=w894, "Force Group Priorities"=w898, "Forces Error \nWindow"=w899, "Mixed Mode Convergence Status In"=w897) -> ("Mixed Mode Convergence Status Out"=w901:T22)  [unwired: 5 in, 1 out]
          n451 = Unbundle By Name(w901) -> ("IsConverged"=w896:bool[])
          n452 = call "Convergence Status DAO.vi"("Convergence Status In"=w901, "LBCB Selected"=w893, "Actions"=DAO_Actions."Set") -> ("Convergence Status Out"=w895:T22)  [unwired: 1 in, 7 out]
        }
        n453 = And Array Elements(Boolean array=w879) -> (logical AND=w892:bool)
        n454 = local write "Convergence Status"(w878) -> ()
        n455 = Select(t=Mixed_Mode_States."Start Stabilize" ("MixedModeStates"), s=w892, f=Mixed_Mode_States."Update Command" ("t")) -> (s? t:f=w884:T23)
      }
      frame "Update Stiffness Jacobian" {
        n456 = local read "Convergence Status"() -> (w924:T22[])
        n457 = Build Array(MM_Result_Actions."Nop" ("MM Result Actions")) -> (w921:T1[])
        n458 = local read "Hold Data"() -> (w918:T7[])
        n459 = local read "Stiffness Limits"() -> (w920:dbl[][][])
        n460 = for {
          tunnel: T12 {"Displacements"=[], "Forces"=[]} ("Increments") -> [w951]
          tunnel: [w940] -> w925 mode=indexing
          tunnel: w924 -> [w944] mode=indexing
          tunnel: w918 -> [w942] mode=indexing
          tunnel: w923 -> [w941] mode=indexing
          tunnel: w920 -> [w939] mode=indexing
          tunnel: [w936] -> w915 mode=indexing
          tunnel: [w935] -> w914 mode=indexing
          i -> [w938]
          n461 = Unbundle By Name(w941) -> ("Displacement \nCommands"=w949:dbl[], "Forces"=w947:dbl[])
          n462 = Unbundle By Name(w942) -> ("Forces"=w943:dbl[], "Displacement \nCommands"=w937:dbl[])
          n463 = Subtract(x=w943, y=w947) -> (x-y=w946:dbl[])
          n464 = Subtract(x=w937, y=w949) -> (x-y=w948:dbl[])
          n465 = call "Calculated Stiffness Jacobian.vi"("LBCB Number"=w938, "Actions"=Persistant_DAO_Actions."Get" ("Stiffness Jacobian Datastore Actions")) -> ("Stiffness Jacobian Out"=w954:T21)  [unwired: 2 in, 7 out]
          n466 = Bundle By Name(cluster=w951, "Displacements"=w948, "Forces"=w946) -> (w950:T12)
          n467 = call "Update Stiffness Jacobian.vi"("Stiffness Limit"=w939, "Mixed Mode Convergence Status In"=w944, "Increments"=w950, "Stiffness Jacobian In"=w954) -> ("Jacobian Stiffness Column"=w936:T3, "Stiffness Jacobian Out"=w953:T21, "Updated"=w935:bool)  [unwired: 5 out]
          n468 = call "Calculated Stiffness Jacobian.vi"("Stiffness Jacobian In"=w953, "LBCB Number"=w938, "Actions"=Persistant_DAO_Actions."Set" ("Stiffness Jacobian Datastore Actions")) -> ("Stiffness Jacobian Out"=w945:T21)  [unwired: 1 in, 7 out]
          n469 = Bundle("Stiffness Jacobian Out"=w945) -> (w940:cluster{"Stiffness Jacobian Out":T21})  [unwired: 1 in]
        }
        n470 = Or Array Elements(Boolean array=w914) -> (logical OR=w913:bool)
        n471 = case shown="True" w913 {
          tunnel: w912 -> [w931 w934]
          tunnel: [w931 w932] -> w911
          frame False {
          }
          frame True {
            n472 = Enqueue Element(queue=w934, element=Command_or_Stiffness_Updates."Stiffness Update") -> (queue out=w932:refnum<queue>)  [unwired: 2 in, 2 out]
          }
        }
        n473 = local write "Stiffness Jacobian Column"(w915) -> ()
        n474 = local write "Stiffness Jacobian"(w925) -> ()
      }
      frame "Update Command" {
        w971 = DAO_Actions."Get" ("Mixed Mode Commands\n Datastore Actions")
        n475 = local read "Hold Data"() -> (w961:T7[])
        n476 = call "Mixed Mode Commands DAO.vi"("Mixed Mode Commands\n Datastore Actions"=w971) -> ("Current Target"=w974:T5[])  [unwired: 3 in, 7 out]
        n477 = Build Array(MM_Result_Actions."Nop" ("MM Result Actions")) -> (w963:T1[])
        n478 = local read "Max Increment"() -> (w965:dbl[][])
        n479 = local read "Jacobian Gain"() -> (w966:dbl[][])
        n480 = for {
          tunnel: w974 -> [w979] mode=indexing
          tunnel: w971 -> [w990]
          tunnel: [w987] -> w970 mode=indexing
          tunnel: w967 -> [w982] mode=indexing
          tunnel: w966 -> [w986] mode=indexing
          tunnel: w965 -> [w985] mode=indexing
          tunnel: w961 -> [w984] mode=indexing
          tunnel: w958 -> [w978] mode=indexing
          n481 = Unbundle By Name(w984) -> ("Forces"=w977:dbl[])
          n482 = call "Calculated Stiffness Jacobian.vi"("LBCB Number"=w982, "Actions"=Persistant_DAO_Actions."Get") -> ("Stiffness Jacobian Out"=w980:T21)  [unwired: 8 in, 1 out]
          n483 = call "Convergence Status DAO.vi"("LBCB Selected"=w982, "Actions"=w990) -> ("Convergence Status Out"=w983:T22)  [unwired: 2 in, 7 out]
          n484 = Unbundle By Name(w983) -> ("IsConverged"=w989:bool[])
          n485 = And Array Elements(Boolean array=w989) -> (logical AND=w988:bool)
          n486 = case shown="True" w988 {
            tunnel: [w995 w999] -> w987
            tunnel: w979 -> [w996 w1000]
            tunnel: w977 -> [w991 _]
            tunnel: w986 -> [w993 _]
            tunnel: w985 -> [w994 _]
            tunnel: w983 -> [w997 _]
            tunnel: w980 -> [w992 _]
            tunnel: w978 -> [_ w998]
            frame False {
              n487 = call "Update Iterative Command.vi"("Stiffness Jacobian In"=w992, "Maximum Displacement\nIncrement"=w994, "Jacobian Gain"=w993, "Convergence Status In"=w997, "Current Forces"=w991, "Target  Command Data In"=w996) -> ("Updated  Command Data Out"=w995:T5)  [unwired: 5 in]
            }
            frame True {
              n488 = call "Command Data 2 Control Target.vi"("Current Command"=w998, "Current Target"=w1000) -> ("Output"=w999:T5)  [unwired: 1 in, 8 out]
            }
          }
        }
        n489 = call "Mixed Mode Commands DAO.vi"("Current Target In"=w970, "Mixed Mode Commands\n Datastore Actions"=DAO_Actions."Set" ("Mixed Mode Commands\n Datastore Actions")) -> ("Current Target"=w969:T5[])  [unwired: 3 in, 6 out]
        n490 = local write "Iterative Target"(w969) -> ()
      }
      frame "Start Iterative Ramp" {
        w1008 = T1[] [enum."Check Limits", enum."Store Prev Reading", enum."Hold Off", enum."Averaging Off"] items=["Nop", "Set Command", "Check Limits", "Send Command", "Store Prev Reading", "Averaging On", "Averaging Off", "Hold On", "Hold Off", "PID Hold On", "PID Hold Off", "Clear Increment Faults", "Set Initial Position"]
        n491 = Unbundle By Name(w1009) -> ("Ramp Times.Iterative"=w1017:T31)
        n492 = Unbundle By Name(w1017) -> ("Ramp"=w1013:dbl)
        n493 = Equal To 0?(x=w1013) -> (x = 0?=w1014:bool)
        n494 = Select(t=0.1, s=w1014, f=w1013) -> (s? t:f=w1012:dbl)
        n495 = Enqueue Element(queue=w1004, element=Command_or_Stiffness_Updates."Iterative Command Update") -> (queue out=w1003:refnum<queue>)  [unwired: 2 in, 2 out]
        n496 = Bundle By Name(cluster=w1017, "Ramp"=w1012) -> (w1015:T31)
      }
      frame "Run Iterative Ramp" {
        w1027 = T1[] [enum."Set Command", enum."Check Limits", enum."Send Command"] items=["Nop", "Set Command", "Check Limits", "Send Command", "Store Prev Reading", "Averaging On", "Averaging Off", "Hold On", "Hold Off", "PID Hold On", "PID Hold Off", "Clear Increment Faults", "Set Initial Position"]
        n497 = call "Ramp Time Completions.vi"("Current Ramp Time"=w1039, "Initial"=w1037) -> ("Still in Ramp"=w1040:bool, "Fraction\nCompleted"=w1041:dbl)
        n498 = case shown="False" w1040 {
          tunnel: w1041 -> [_ w1048]
          tunnel: [Mixed_Mode_States."Start Iterative Stabilize" ("MixedModeStates") Mixed_Mode_States."Run Iterative Ramp" ("MixedModeStates")] -> w1026
          tunnel: [w1043 w1046] -> w1021
          frame False {
            n499 = call "Mixed Mode Commands DAO.vi"("Mixed Mode Commands\n Datastore Actions"=DAO_Actions."Get" ("Mixed Mode Commands\n Datastore Actions")) -> ("Current Target"=w1043:T5[])  [unwired: 3 in, 7 out]
          }
          frame True {
            n500 = call "Calculate Ramp Displacements.vi"("Iterative\nRamp"=TRUE ("Iterative\nRamp"), "Ramp Time"=w1048) -> ("Target"=w1046:T5[])  [unwired: 1 in]
          }
        }
        n501 = Dequeue Element(queue=w1034, timeout in ms (-1)=w1029) -> (queue out=w1033:refnum<queue>, element=w1035:T34, timed out?=w1036:bool)  [unwired: 1 in, 1 out]
        n502 = Select(t=w1032, s=w1036, f=w1035) -> (s? t:f=w1031:T34)
        n503 = local write "Target"(w1021) -> ()
        n504 = call "MM Command to Cntrl Loop Actuator In.vi"("Target"=w1021, "Current Cartesian Position"=w1023, "Number of\nLBCBs In"=w1030, "error in (no error)"=w1019, "Rigid Connection"=w1020) -> ("Cmd Out"=w1028:T2[], "error out"=w1018:errorcluster)  [unwired: 6 in, 3 out]
      }
      frame "Start Iterative Stabilize" {
        w1054 = T1[] [enum."Averaging On", enum."Check Limits"] items=["Nop", "Set Command", "Check Limits", "Send Command", "Store Prev Reading", "Averaging On", "Averaging Off", "Hold On", "Hold Off", "PID Hold On", "PID Hold Off", "Clear Increment Faults", "Set Initial Position"]
        n505 = Unbundle By Name(w1055) -> ("Ramp Times.Iterative"=w1057:T31)
      }
      frame "Iterative Stabilize" {
        w1064 = T1[] [enum."Averaging On", enum."Check Limits"] items=["Nop", "Set Command", "Check Limits", "Send Command", "Store Prev Reading", "Averaging On", "Averaging Off", "Hold On", "Hold Off", "PID Hold On", "PID Hold Off", "Clear Increment Faults", "Set Initial Position"]
        n506 = Unbundle By Name(w1072) -> ("Stab"=w1077:dbl)
        n507 = Divide(x=w1074, y=u64 1000) -> (x/y=w1076:dbl)
        n508 = Greater?(x=w1076, y=w1077) -> (0:w1073:bool)
        n509 = Dequeue Element(queue=w1069, timeout in ms (-1)=w1065) -> (queue out=w1068:refnum<queue>, element=w1070:T34, timed out?=w1071:bool)  [unwired: 1 in, 1 out]
        n510 = Select(t=w1067, s=w1071, f=w1070) -> (s? t:f=w1066:T34)
        n511 = Select(t=Mixed_Mode_States."Start Iterative Holding" ("MixedModeStates"), s=w1073, f=Mixed_Mode_States."Iterative Stabilize" ("MixedModeStates")) -> (s? t:f=w1063:T23)
      }
      frame "Start Iterative Holding" {
        w1086 = T1[] [enum."Averaging On", enum."Hold On", enum."Check Limits"] items=["Nop", "Set Command", "Check Limits", "Send Command", "Store Prev Reading", "Averaging On", "Averaging Off", "Hold On", "Hold Off", "PID Hold On", "PID Hold Off", "Clear Increment Faults", "Set Initial Position"]
      }
      frame "Iterative Holding" {
        w1096 = T1[] [enum."Averaging On", enum."Hold On", enum."Check Limits"] items=["Nop", "Set Command", "Check Limits", "Send Command", "Store Prev Reading", "Averaging On", "Averaging Off", "Hold On", "Hold Off", "PID Hold On", "PID Hold Off", "Clear Increment Faults", "Set Initial Position"]
        n512 = Divide(x=w1106, y=u64 1000) -> (x/y=w1108:dbl)
        n513 = Unbundle By Name(w1109) -> ("Hold"=w1105:dbl)
        n514 = Greater?(x=w1108, y=w1105) -> (0:w1104:bool)
        n515 = Dequeue Element(queue=w1101, timeout in ms (-1)=w1097) -> (queue out=w1100:refnum<queue>, element=w1102:T34, timed out?=w1103:bool)  [unwired: 1 in, 1 out]
        n516 = Select(t=w1099, s=w1103, f=w1102) -> (s? t:f=w1098:T34)
        n517 = Select(t=Mixed_Mode_States."Update Stiffness Jacobian" ("MixedModeStates"), s=w1104, f=Mixed_Mode_States."Iterative Holding") -> (s? t:f=w1095:T23)
      }
      frame "Start Stabilize" {
        w1118 = T1[] [enum."Averaging On", enum."Check Limits", enum."PID Hold On"] items=["Nop", "Set Command", "Check Limits", "Send Command", "Store Prev Reading", "Averaging On", "Averaging Off", "Hold On", "Hold Off", "PID Hold On", "PID Hold Off", "Clear Increment Faults", "Set Initial Position"]
        n518 = Unbundle By Name(w1119) -> ("Ramp Times.Initial"=w1121:T31)
      }
      frame "Stabilize" {
        w1128 = T1[] [enum."Averaging On", enum."Check Limits", enum."PID Hold On"] items=["Nop", "Set Command", "Check Limits", "Send Command", "Store Prev Reading", "Averaging On", "Averaging Off", "Hold On", "Hold Off", "PID Hold On", "PID Hold Off", "Clear Increment Faults", "Set Initial Position"]
        n519 = Unbundle By Name(w1136) -> ("Stab"=w1141:dbl)
        n520 = Divide(x=w1138, y=u64 1000) -> (x/y=w1140:dbl)
        n521 = Dequeue Element(queue=w1133, timeout in ms (-1)=w1129) -> (queue out=w1132:refnum<queue>, element=w1134:T34, timed out?=w1135:bool)  [unwired: 1 in, 1 out]
        n522 = Greater?(x=w1140, y=w1141) -> (0:w1137:bool)
        n523 = Select(t=w1131, s=w1135, f=w1134) -> (s? t:f=w1130:T34)
        n524 = Select(t=Mixed_Mode_States."Start Hold" ("MixedModeStates"), s=w1137, f=Mixed_Mode_States."Stabilize" ("MixedModeStates")) -> (s? t:f=w1127:T23)
      }
      frame "Start Hold" {
        w1150 = T1[] [enum."Averaging On", enum."Check Limits", enum."PID Hold On", enum."Hold On"] items=["Nop", "Set Command", "Check Limits", "Send Command", "Store Prev Reading", "Averaging On", "Averaging Off", "Hold On", "Hold Off", "PID Hold On", "PID Hold Off", "Clear Increment Faults", "Set Initial Position"]
      }
      frame "Holding" {
        w1160 = T1[] [enum."Averaging On", enum."Check Limits", enum."PID Hold On", enum."Hold On"] items=["Nop", "Set Command", "Check Limits", "Send Command", "Store Prev Reading", "Averaging On", "Averaging Off", "Hold On", "Hold Off", "PID Hold On", "PID Hold Off", "Clear Increment Faults", "Set Initial Position"]
        n525 = Unbundle By Name(w1173) -> ("Hold"=w1169:dbl)
        n526 = Divide(x=w1170, y=u64 1000) -> (x/y=w1172:dbl)
        n527 = Greater?(x=w1172, y=w1169) -> (0:w1168:bool)
        n528 = Dequeue Element(queue=w1165, timeout in ms (-1)=w1161) -> (queue out=w1164:refnum<queue>, element=w1166:T34, timed out?=w1167:bool)  [unwired: 1 in, 1 out]
        n529 = Select(t=w1163, s=w1167, f=w1166) -> (s? t:f=w1162:T34)
        n530 = Select(t=Mixed_Mode_States."Done" ("MixedModeStates"), s=w1168, f=Mixed_Mode_States."Holding") -> (s? t:f=w1159:T23)
      }
      frame "Done" {
        w1183 = T1[] [enum."Averaging Off", enum."Hold Off", enum."PID Hold Off"] items=["Nop", "Set Command", "Check Limits", "Send Command", "Store Prev Reading", "Averaging On", "Averaging Off", "Hold On", "Hold Off", "PID Hold On", "PID Hold Off", "Clear Increment Faults", "Set Initial Position"]
        n531 = Wait Until Next ms Multiple(millisecond multiple=w1181) -> ()  [unwired: 1 out]
      }
      frame "Exit" {
        w1192 = T1[] [enum."Averaging Off", enum."Hold Off", enum."PID Hold Off"] items=["Nop", "Set Command", "Check Limits", "Send Command", "Store Prev Reading", "Averaging On", "Averaging Off", "Hold On", "Hold Off", "PID Hold On", "PID Hold Off", "Clear Increment Faults", "Set Initial Position"]
      }
      frame "Nop" {
        n532 = Build Array(MM_Result_Actions."Nop" ("MM Result Actions")) -> (w1202:T1[])
      }
    }
    n533 = for {
      tunnel: w524 -> [w1223] mode=indexing
      tunnel: w543 -> [w1222] mode=indexing
      tunnel: [w1221] -> w544 mode=indexing
      n534 = Bundle By Name(cluster=w1222, "Act Cmd"=w1223) -> (w1221:T2)
    }
    n535 = Equal?(x=w551, y=w550) -> (x = y?=w552:bool)
    n536 = Array Size(array=w547) -> (size(s)=w546:i32)
    n537 = while {
      shift-right: [w1250] -> w577
      shift-left: w545 -> [w1235]
      shift-right: [w1249] -> w576
      shift-left: w544 -> [w1248]
      tunnel: w547 -> [w1247] mode=indexing
      shift-right: [w1246] -> w575
      shift-left: w572 -> [w1245]
      tunnel: w574 -> [w1244]
      shift-right: [w1240] -> w560
      shift-left: w571 -> [w1243]
      shift-right: [w1239] -> w561
      shift-left: w570 -> [w1242]
      shift-right: [w1238] -> w562
      shift-left: w569 -> [w1241]
      shift-right: [w1237] -> w558
      shift-left: w559 -> [w1236]
      shift-right: [w1234] -> w549
      shift-left: w548 -> [w1233]
      tunnel: w536 -> [w1232]
      tunnel: w546 -> [w1228]
      tunnel: w542 -> [w1226]
      shift-right: [w1224] -> w517
      shift-left: w521 -> [w1225]
      i -> [w1229]
      stop <- w1231 stop-if-true
      # "Previous\nReading"
      # "Measurements"
      # "Current \nCommands"
      # "Previous\nCommands"
      # "Limits Check"
      n538 = local write "MM Result Actions"(w1247) -> ()
      n539 = case shown="\"Check Limits\"" w1247 {
        tunnel: [w1253 w1272 w1279 w1288 w1297 w1306 w1315 w1324 w1342 w1357 w1372 w1382 w1393] -> w1250
        tunnel: [w1259 w1264 w1283 w1293 w1302 w1311 w1320 w1328 w1347 w1351 w1371 w1381 w1398] -> w1249
        tunnel: w1248 -> [w1259 w1274 w1283 w1293 w1302 w1311 w1320 w1328 w1347 w1354 w1369 w1381 w1398]
        tunnel: [w1258 w1273 w1284 w1294 w1303 w1312 w1321 w1329 w1348 w1358 w1373 w1383 w1391] -> w1246
        tunnel: w1245 -> [w1258 w1273 w1284 w1294 w1303 w1312 w1321 w1329 w1348 w1358 w1373 w1383 _]
        tunnel: w1244 -> [_ _ _ _ _ _ _ _ _ w1351 w1371 _ _]
        tunnel: [w1257 w1271 TRUE w1291 w1301 w1310 w1318 FALSE w1346 w1361 w1376 w1386 w1397] -> w1240
        tunnel: w1243 -> [w1257 w1271 _ w1291 w1301 w1310 w1318 _ w1346 w1361 w1376 w1386 w1397]
        tunnel: [w1256 w1270 w1282 TRUE w1300 w1309 FALSE w1327 w1345 w1360 w1375 w1385 w1396] -> w1239
        tunnel: w1242 -> [w1256 w1270 w1282 _ w1300 w1309 _ w1327 w1345 w1360 w1375 w1385 w1396]
        tunnel: [w1255 w1269 w1281 w1290 TRUE FALSE w1317 w1326 w1344 w1359 w1374 w1384 w1395] -> w1238
        tunnel: w1241 -> [w1255 w1269 w1281 w1290 _ _ w1317 w1326 w1344 w1359 w1374 w1384 w1395]
        tunnel: [w1254 w1266 w1280 w1289 w1298 w1307 w1316 w1325 w1343 w1353 w1370 w1378 w1394] -> w1237
        tunnel: w1236 -> [w1254 w1265 w1280 w1289 w1298 w1307 w1316 w1325 w1343 w1355 w1370 w1379 w1394]
        tunnel: w1235 -> [w1253 w1263 w1279 w1288 w1297 w1306 w1315 w1324 w1342 w1357 w1372 w1382 w1393]
        tunnel: [w1252 w1268 w1278 w1287 w1296 w1305 w1314 w1323 w1341 w1350 w1369 w1380 w1392] -> w1234
        tunnel: w1233 -> [w1252 w1268 w1278 w1287 w1296 w1305 w1314 w1323 w1341 w1350 _ w1380 w1392]
        tunnel: w1232 -> [_ w1262 _ _ _ _ _ _ _ _ _ _ _]
        tunnel: [_ w1267 _ _ _ _ _ _ _ _ _ _ _] -> w1230
        tunnel: w1226 -> [_ _ _ _ _ _ _ _ _ w1352 _ _ _]
        tunnel: w1225 -> [w1251 w1261 w1277 w1286 w1295 w1304 w1313 w1322 w1331 w1349 w1368 w1377 w1390]
        tunnel: [w1251 w1260 w1277 w1286 w1295 w1304 w1313 w1322 w1331 w1349 w1368 w1377 w1390] -> w1224
        frame "Nop" {
        }
        frame "Check Limits" {
          # "For Rigid Connection Forces and Displacements\nare checked with individual LBCB readings then \ncombined"
          # "We set commands\nhere even during an abort because\nwe want to show what the exceeded \nlimits are"
          # "Collect Measurements and Check Limits"
          n540 = local read "Actuator Meas. Disp & Forces"() -> (w1276:dbl[][])
          n541 = local read "Limits"() -> (w1275:T18[])
          n542 = flat-sequence {
            tunnel: w1263 -> [_]
            frame #0 {
            }
          }
          n543 = call "Collect All Measurements.vi"("Limits"=w1275, "Rigid Connection"=w1262, "error in (no error)"=w1261, "Actuator Meas. Disp & Forces"=w1276, "Cmd In"=w1274, "Within Limits In"=w1265) -> ("error out"=w1260:errorcluster, "Within Limits Out"=w1266:T14[], "Measurements Out"=w1272:T20[], "Cmds Out"=w1264:T2[])  [unwired: 2 in]
          n544 = call "Check For Abort.vi"("Within Limits"=w1266) -> ("Faulted"=w1267:bool)  [unwired: 1 in, 1 out]
          n545 = local write "Commands"(w1264) -> ()
          n546 = local write "Limits Check"(w1266) -> ()
          n547 = local write "Measurements"(w1272) -> ()
        }
        frame "Averaging On" {
        }
        frame "Hold On" {
        }
        frame "PID Hold On" {
        }
        frame "PID Hold Off" {
        }
        frame "Hold Off" {
        }
        frame "Averaging Off" {
        }
        frame "Send Command" {
          n548 = Index Array(array=w1347, index #1=0 ("index"), index #2=1 ("index")) -> (element #1=w1339:T2, element #2=w1336:T2)
          n549 = Unbundle By Name(w1339) -> ("Act Cmd"=w1340:dbl[], "Cart Cmd"=w1333:dbl[])
          n550 = Unbundle By Name(w1336) -> ("Act Cmd"=w1335:dbl[], "Cart Cmd"=w1332:dbl[])
          n551 = local write "L1 Ctrl Loop In Actuator"(w1340) -> ()
          n552 = local write "L2 Ctrl Loop In Actuator"(w1335) -> ()
          n553 = call "Current Position DAO.vi"("LBCB 2 Commands In"=w1332, "LBCB 1 Commands In"=w1333, "Actions"=DAO_Actions."Set") -> ()  [unwired: 7 in, 2 out]
        }
        frame "Set Command" {
          # "\"Set Command\" is supposed to be followed by\n\"Check Limits\".  At that point an increment fault\nwill abort the command"
          n554 = local read "Increment Limits"() -> (w1356:T2[])
          n555 = for {
            tunnel: w1356 -> [w1367] mode=indexing
            tunnel: w1355 -> [w1366] mode=indexing
            tunnel: w1351 -> [w1362] mode=indexing
            tunnel: w1354 -> [w1365] mode=indexing
            tunnel: [w1364] -> w1353 mode=indexing
            tunnel: w1352 -> [w1363] mode=indexing
            n556 = call "Calculate Increment.vi"("LBCB Number"=w1363, "Increment Limits"=w1367, "Previous"=w1365, "Current"=w1362, "Within Limits In"=w1366) -> ("Within Limits Out"=w1364:T14)  [unwired: 5 in, 1 out]
          }
        }
        frame "Set Initial Position" {
        }
        frame "Clear Increment Faults" {
          n557 = for {
            tunnel: w1379 -> [w1389] mode=indexing
            tunnel: [w1388] -> w1378 mode=indexing
            w1387 = TRUE ("Increments.Dx")
            n558 = Bundle By Name(cluster=w1389, "Act Incr.X1"=w1387, "Act Incr.X2"=w1387, "Act Incr.Y1"=w1387, "Act Incr.Z1"=w1387, "Act Incr.Z2"=w1387, "Act Incr.Z3"=w1387, "Cart Incr.Dx"=w1387, "Cart Incr.Dy"=w1387, "Cart Incr.Dz"=w1387, "Cart Incr.Rx"=w1387, "Cart Incr.Ry"=w1387, "Cart Incr.Rz"=w1387) -> (w1388:T14)
          }
        }
        frame "Store Prev Reading" {
          # "Store for Stiffness\nJacobian Previous Target"
          n559 = local read "Hold Data"() -> (w1391:T7[])
        }
      }
      n560 = Greater Or Equal?(x=w1229, y=w1228) -> (x >= y?=w1227:bool)
      n561 = Or(x=w1230, y=w1227) -> (x .or. y?=w1231:bool)
    }
    "Collecting DAQ Samples" <- w560
    n562 = case shown="True" w552 {
      tunnel: w555 -> [w1400 w1405]
      tunnel: [w1400 w1404] -> w554
      tunnel: w521 -> [w1399 w1403]
      tunnel: [w1399 w1402] -> w553
      tunnel: w551 -> [_ w1401]
      frame False {
      }
      frame True {
        n563 = Enqueue Element(queue=w1405, element=w1401, error in (no error)=w1403) -> (queue out=w1404:refnum<queue>, error out=w1402:errorcluster)  [unwired: 1 in, 1 out]
      }
    }
    n564 = call "GetSamplingRate.vi"() -> ("Sampling"=w580:i32)
    n565 = local write "Mixed Mode"(w580) -> ()
    n566 = local read "PID Control"() -> (w563:T24[])
    n567 = Merge Errors(w519, w517, w553) -> (w520:errorcluster)
    n568 = case shown="\"Start Initial Ramp\", Default" w551 {
      tunnel: w558 -> [_ _ _ _ _ _ _ w1218 _ _]
      tunnel: [w1209 w1210 w1211 w1212 w1213 w1214 w1215 w1217 w1219 w1220] -> w557
      tunnel: w556 -> [w1209 w1210 w1211 w1212 w1213 w1214 w1215 w1216 w1219 w1220]
      frame "Aborting" {
      }
      frame "Exit" {
      }
      frame "Nop" {
      }
      frame "Wait For DAQ" {
      }
      frame "Idle" {
      }
      frame "Start Initial Position" {
      }
      frame "Initial Position" {
      }
      frame "Start Initial Ramp", Default {
        n569 = call "Check For Abort.vi"("Mixed Mode State In"=w1216, "Within Limits"=w1218) -> ("Mixed Mode State Out"=w1217:T23)  [unwired: 1 out]
      }
      frame "Init" {
      }
      frame "Done" {
      }
    }
    n570 = for {
      tunnel: [w1408] -> w564 mode=indexing
      tunnel: w563 -> [w1407] mode=indexing
      tunnel: w562 -> [w1406]
      n571 = Unbundle By Name(w1407) -> ("I-Control"=w1410:bool, "Ctrl Mode"=w1409:bool)
      n572 = Compound Arithmetic op=AND(w1410, w1409, w1406) -> (w1408:bool)
    }
    n573 = call "Error Logger.vi"("error in (no error)"=w520) -> ("error out"=w518:errorcluster)  [unwired: 10 in]
    n574 = Not Equal?(x=w557, y=w551) -> (x != y?=w589:bool)
    n575 = local write "Averaging"(w560) -> ()
    n576 = case shown="True" w589 {
      tunnel: w554 -> [w1412 w1417]
      tunnel: [w1412 w1416] -> w590
      tunnel: w518 -> [w1411 w1415]
      tunnel: [w1411 w1414] -> w585
      tunnel: w557 -> [_ w1413]
      frame False {
      }
      frame True {
        n577 = Enqueue Element(queue=w1417, element=w1413, error in (no error)=w1415) -> (queue out=w1416:refnum<queue>, error out=w1414:errorcluster)  [unwired: 1 in, 1 out]
      }
    }
    n578 = local read "App Running"() -> (w581:bool)
    n579 = local write "MixedModeStates"(w557) -> ()
    n580 = Index Array(array=w564, index #1=0 ("index"), index #2=1 ("index")) -> (element #1=w567:bool, element #2=w568:bool)
    n581 = local write "Hold Period"(w561) -> ()
    n582 = Not(x=w581) -> (.not. x?=w579:bool)
    n583 = local write "L1 PID On"(w567) -> ()
    n584 = local write "L2 PID On"(w568) -> ()
  }
  n585 = call "Autobalance Initial State DAO.vi"() -> ("autobalance\nfile"=w96:string, "Initial Values"=w100:T8[])  [unwired: 3 in, 7 out]
  n586 = Initialize Array(0.0 ("element"), 6 ("dimension size")) -> (w47:dbl[])
  n587 = call "Autobalance Initial State DAO.vi"() -> ("Initial Values"=w95:T8[])  [unwired: 3 in, 8 out]
  n588 = while {
    shift-right: [w1437] -> _
    shift-left: w47 -> [w1440]
    tunnel: w73 -> [w1439]
    shift-right: [w1432] -> _
    shift-left: w100 -> [w1435]
    tunnel: LBCB_Number."LBCB1" ("LBCB Number") -> [w1434]
    tunnel: [w1433] -> w92
    shift-right: [w1431] -> _
    shift-left: Autobalance_State."Init" ("Autobalance State Out") -> [w1430]
    shift-right: [w1429] -> _
    shift-left: _ -> [w1428]
    shift-right: [w1427] -> _
    shift-left: _ -> [w1426]
    tunnel: w61 -> [w1425]
    stop <- w1433 stop-if-true
    # "LBCB 1 Control Loop"
    # "Cartesian\nCommand\nNo  Offset"
    # "Actuator Command"
    n589 = local read "L1 Ctrl Loop In Actuator"() -> (w1424:dbl[])
    n590 = call "GetSamplingRate.vi"() -> ("Sampling"=w1438:i32)
    n591 = local read "App Running"() -> (w1441:bool)
    n592 = local read "L1 Ctrl Loop State"() -> (w1442:T13)
    n593 = local write "L1 Control Rate"(w1438) -> ()
    n594 = Not(x=w1441) -> (.not. x?=w1433:bool)
    n595 = case shown="\"On\"" w1442 {
      tunnel: w1438 -> [_ _ _ _ _ _ _]
      tunnel: [w1447 w1453 w1461 w1463 w1498 w1508 w1511] -> w1437
      tunnel: w1440 -> [w1447 w1453 w1461 _ _ w1508 _]
      tunnel: w1439 -> [w1448 w1454 w1462 w1474 w1497 w1509 w1517]
      tunnel: w1434 -> [_ _ _ w1468 w1496 _ w1516]
      tunnel: w1424 -> [_ _ _ _ _ _ w1511]
      tunnel: [w1446 w1452 w1460 w1472 w1491 w1507 w1515] -> w1427
      tunnel: [w1449 w1455 w1458 w1464 w1488 w1510 w1514] -> w1432
      tunnel: w1435 -> [w1449 w1455 _ w1465 w1489 w1510 w1514]
      tunnel: [w1445 w1451 Autobalance_State."Init" ("Autobalance State Out") w1467 w1494 w1506 w1513] -> w1431
      tunnel: w1430 -> [w1445 w1451 _ w1467 w1495 w1506 w1513]
      tunnel: [w1444 w1450 T9 TRUE ("InitialPosition? Out") w1466 w1492 w1505 w1512] -> w1429
      tunnel: w1428 -> [w1444 w1450 _ w1466 w1493 w1505 w1512]
      tunnel: w1426 -> [_ _ _ _ w1490 _ _]
      tunnel: w1425 -> [_ _ _ _ w1484 _ _]
      frame "Idle" {
        n596 = Wait Until Next ms Multiple(millisecond multiple=u32 1000) -> ()  [unwired: 1 out]
        n597 = Divide(x=w1447, y=w1448) -> (x/y=w1446:dbl[])
      }
      frame "Off" {
        n598 = Divide(x=w1453, y=w1454) -> (x/y=w1452:dbl[])
      }
      frame "Reset Autobalancing" {
        n599 = call "Autobalance Initial State DAO.vi"() -> ("Initial Values"=w1458:T8[])  [unwired: 2 in, 9 out]
        n600 = local write "L1 Ctrl Loop State"(Control_Loop_State."Autobalancing" ("L1 Ctrl Loop State")) -> ()
        n601 = Divide(x=w1461, y=w1462) -> (x/y=w1460:dbl[])
      }
      frame "Set Command" {
        n602 = call "Initial Command DAO.vi"("LBCB Number"=w1468, "DAO Actions"=DAO_Actions."Get") -> ("Command Out"=w1470:T41)  [unwired: 2 in, 7 out]
        n603 = call "Actuator Point 2 Array.vi"("Actuator Point"=w1470) -> ("Array"=w1463:dbl[])
        n604 = for {
          tunnel: w1465 -> [w1477] mode=indexing
          tunnel: [w1475] -> w1464 mode=indexing
          n605 = Bundle By Name(cluster=w1477, "IsBalanced"=T9 TRUE) -> (w1475:T8)
        }
        n606 = local write "L1 Ctrl Loop In Actuator"(w1463) -> ()
        n607 = local write "L1 Ctrl Loop State"(Control_Loop_State."Ready for Control" ("L1 Ctrl Loop State")) -> ()
        n608 = Divide(x=w1463, y=w1474) -> (x/y=w1472:dbl[])
        n609 = call "Daq Send.vi"("LBCB Select"=w1468, "Commands"=w1472, "Daq Actions"=Daq_Actions."Send Commands") -> ()  [unwired: 2 in, 7 out]
      }
      frame "Autobalancing" {
        n610 = local read "Auto Balance Error Tolerance"() -> (w1482:dbl[][])
        n611 = local read "Servo Error"() -> (w1485:dbl[][])
        n612 = Index Array(array=w1485, index (row)=0 ("disabled index (col)")) -> (element=w1483:dbl[])  [unwired: 1 in]
        n613 = local read "AB Parameters"() -> (w1478:T6)
        n614 = Subtract(x=w1483, y=w1484) -> (x-y=w1486:dbl[])
        n615 = Index Array(array=w1482, index (row)=0 ("disabled index (col)")) -> (element=w1481:dbl[])  [unwired: 1 in]
        n616 = call "Autobalance.vi"("Servo Errors"=w1486, 1:"Autobalance State In"=w1495, "LBCB Number"=w1496, "InitialPosition? In"=w1493, "Error Tolerance"=w1481, "Command In"=w1490, 11:"Autobalance State In"=w1489, "Autobalance \nControl Parameters"=w1478) -> ("IsBalanced"=w1487:T9, "Command Out"=w1491:dbl[], "InitialPosition? Out"=w1492:T9, 14:"Autobalance State Out"=w1494:T30, 15:"Autobalance State Out"=w1488:T8[])  [unwired: 3 out]
        n617 = Multiply(x=w1497, y=w1491) -> (x*y=w1498:dbl[])
        n618 = case shown="True" w1487 {
          tunnel: w1498 -> [_ w1503]
          tunnel: w1496 -> [_ w1501]
          frame False {
          }
          frame True {
            n619 = call "Array 2 Actuator Point.vi"("Array"=w1503) -> ("Actuator Point"=w1504:T41)
            n620 = local write "L1 Ctrl Loop State"(Control_Loop_State."Set Command" ("L1 Ctrl Loop State")) -> ()
            n621 = call "Initial Command DAO.vi"("Command In"=w1504, "LBCB Number"=w1501, "DAO Actions"=DAO_Actions."Set") -> ()  [unwired: 1 in, 8 out]
          }
        }
        n622 = call "Daq Send.vi"("LBCB Select"=w1496, "Commands"=w1491, "Daq Actions"=Daq_Actions."Send Commands") -> ()  [unwired: 2 in, 7 out]
      }
      frame "Ready for Control" {
        n623 = Divide(x=w1508, y=w1509) -> (x/y=w1507:dbl[])
      }
      frame "On" {
        # "4. Actiator and Cartesian Limit Check"
        # "3. Actuator to Cartesian, Cartesian to Actuator Conversions"
        n624 = Divide(x=w1511, y=w1517) -> (x/y=w1515:dbl[])
        n625 = call "Daq Send.vi"("LBCB Select"=w1516, "Commands"=w1515, "Daq Actions"=Daq_Actions."Send Commands") -> ()  [unwired: 2 in, 7 out]
      }
    }
    n626 = local write "L1 Ctrl Loop Out Actuator"(w1437) -> ()
    n627 = local write "L1 Autobalance Out"(w1432) -> ()
    n628 = local write "L1 Cmd  Volts"(w1427) -> ()
    n629 = Wait Until Next ms Multiple(millisecond multiple=u32 4) -> ()  [unwired: 1 out]
  }
  n630 = while {
    tunnel: [w1528] -> _
    shift-right: [w1533] -> _
    shift-left: _ -> [w1535]
    tunnel: w68 -> [w1534]
    shift-right: [w1527] -> _
    shift-left: w95 -> [w1532]
    tunnel: LBCB_Number."LBCB2" ("LBCB Number") -> [w1530]
    tunnel: [w1528] -> w91
    shift-right: [w1526] -> _
    shift-left: _ -> [w1525]
    shift-right: [w1524] -> _
    shift-left: _ -> [w1522]
    shift-right: [w1523] -> _
    shift-left: _ -> [w1521]
    tunnel: w13 -> [_]
    tunnel: w60 -> [w1520]
    stop <- w1528 stop-if-true
    # "LBCB 2 Control Loop"
    # "Cartesian\nCommand\nNo  Offset"
    # "Actuator Command"
    n631 = local read "L2 Ctrl Loop In Actuator"() -> (w1519:dbl[])
    n632 = call "GetSamplingRate.vi"() -> ("Sampling"=w1529:i32)
    n633 = local read "App Running"() -> (w1536:bool)
    n634 = local read "L2 Ctrl Loop State"() -> (w1537:T13)
    n635 = local write "L2 Control Rate"(w1529) -> ()
    n636 = Not(x=w1536) -> (.not. x?=w1528:bool)
    n637 = case shown="\"On\"" w1537 {
      tunnel: w1529 -> [_ _ _ _ _ _ _]
      tunnel: [w1541 w1551 w1558 w1574 w1586 w1604 w1607] -> w1533
      tunnel: w1535 -> [_ w1551 w1558 _ _ w1604 _]
      tunnel: w1534 -> [w1542 w1550 w1559 w1578 w1593 w1605 w1613]
      tunnel: w1530 -> [_ _ _ w1569 w1592 _ w1612]
      tunnel: w1519 -> [w1541 _ _ _ _ _ w1607]
      tunnel: [w1543 w1549 w1557 w1575 w1594 w1606 w1611] -> w1526
      tunnel: [w1544 w1552 w1556 w1577 w1587 w1603 w1610] -> w1527
      tunnel: w1532 -> [w1544 w1552 _ w1579 w1588 w1603 w1610]
      tunnel: w1525 -> [_ _ _ w1573 _ _ _]
      tunnel: [w1540 w1548 T9 TRUE ("InitialPosition? Out") w1572 w1590 w1602 w1609] -> w1524
      tunnel: [w1539 w1547 Autobalance_State."Init" ("Autobalance State Out") w1571 w1589 w1601 w1608] -> w1523
      tunnel: w1522 -> [w1540 w1548 _ w1570 w1590 w1602 w1609]
      tunnel: w1521 -> [w1539 w1547 _ w1568 w1589 w1601 w1608]
      tunnel: w1520 -> [_ _ _ w1566 _ _ _]
      frame "Idle" {
        n638 = Wait Until Next ms Multiple(millisecond multiple=500) -> ()  [unwired: 1 out]
        n639 = Wait Until Next ms Multiple(millisecond multiple=u32 1000) -> ()  [unwired: 1 out]
        n640 = Wait Until Next ms Multiple(millisecond multiple=u32 500) -> ()  [unwired: 1 out]
        n641 = Divide(x=w1541, y=w1542) -> (x/y=w1543:dbl[])
      }
      frame "Off" {
        n642 = Divide(x=w1551, y=w1550) -> (x/y=w1549:dbl[])
      }
      frame "Reset Autobalancing" {
        n643 = local write "L2 Ctrl Loop State"(Control_Loop_State."Autobalancing" ("L1 Ctrl Loop State")) -> ()
        n644 = call "Autobalance Initial State DAO.vi"() -> ("Initial Values"=w1556:T8[])  [unwired: 2 in, 9 out]
        n645 = Divide(x=w1558, y=w1559) -> (x/y=w1557:dbl[])
      }
      frame "Autobalancing" {
        w1561 = 1 ("disabled index (col)")
        n646 = local read "Auto Balance Error Tolerance"() -> (w1565:dbl[][])
        n647 = local read "Servo Error"() -> (w1563:dbl[][])
        n648 = local read "AB Parameters"() -> (w1560:T6)
        n649 = Index Array(array=w1563, index (row)=w1561) -> (element=w1562:dbl[])  [unwired: 1 in]
        n650 = Index Array(array=w1565, index (row)=w1561) -> (element=w1564:dbl[])  [unwired: 1 in]
        n651 = Subtract(x=w1562, y=w1566) -> (x-y=w1567:dbl[])
        n652 = call "Autobalance.vi"("Servo Errors"=w1567, 1:"Autobalance State In"=w1568, "LBCB Number"=w1569, "InitialPosition? In"=w1570, "Error Tolerance"=w1564, "Command In"=w1573, 11:"Autobalance State In"=w1579, "Autobalance \nControl Parameters"=w1560) -> ("IsBalanced"=w1576:T9, "Command Out"=w1575:dbl[], "InitialPosition? Out"=w1572:T9, 14:"Autobalance State Out"=w1571:T30, 15:"Autobalance State Out"=w1577:T8[])  [unwired: 3 out]
        n653 = Multiply(x=w1575, y=w1578) -> (x*y=w1574:dbl[])
        n654 = case shown="True" w1576 {
          tunnel: w1569 -> [_ w1583]
          tunnel: w1574 -> [_ w1582]
          frame False {
          }
          frame True {
            n655 = call "Array 2 Actuator Point.vi"("Array"=w1582) -> ("Actuator Point"=w1584:T41)
            n656 = local write "L2 Ctrl Loop State"(Control_Loop_State."Set Command" ("L1 Ctrl Loop State")) -> ()
            n657 = call "Initial Command DAO.vi"("Command In"=w1584, "LBCB Number"=w1583, "DAO Actions"=DAO_Actions."Set") -> ()  [unwired: 1 in, 8 out]
          }
        }
        n658 = call "Daq Send.vi"("LBCB Select"=w1569, "Commands"=w1575, "Daq Actions"=Daq_Actions."Send Commands") -> ()  [unwired: 2 in, 7 out]
      }
      frame "Set Command" {
        n659 = call "Initial Command DAO.vi"("LBCB Number"=w1592, "DAO Actions"=DAO_Actions."Get") -> ("Command Out"=w1596:T41)  [unwired: 2 in, 7 out]
        n660 = for {
          tunnel: w1588 -> [w1600] mode=indexing
          tunnel: [w1598] -> w1587 mode=indexing
          n661 = Bundle By Name(cluster=w1600, "IsBalanced"=T9 TRUE) -> (w1598:T8)
        }
        n662 = call "Actuator Point 2 Array.vi"("Actuator Point"=w1596) -> ("Array"=w1586:dbl[])
        n663 = local write "L2 Ctrl Loop In Actuator"(w1586) -> ()
        n664 = local write "L2 Ctrl Loop State"(Control_Loop_State."Ready for Control" ("L1 Ctrl Loop State")) -> ()
        n665 = Divide(x=w1586, y=w1593) -> (x/y=w1594:dbl[])
        n666 = call "Daq Send.vi"("LBCB Select"=w1592, "Commands"=w1594, "Daq Actions"=Daq_Actions."Send Commands") -> ()  [unwired: 2 in, 7 out]
      }
      frame "Ready for Control" {
        n667 = Divide(x=w1604, y=w1605) -> (x/y=w1606:dbl[])
      }
      frame "On" {
        # "4. Actiator and Cartesian Limit Check"
        # "3. Actuator to Cartesian, Cartesian to Actuator Conversions"
        n668 = Divide(x=w1607, y=w1613) -> (x/y=w1611:dbl[])
        n669 = call "Daq Send.vi"("LBCB Select"=w1612, "Commands"=w1611, "Daq Actions"=Daq_Actions."Send Commands") -> ()  [unwired: 2 in, 7 out]
      }
    }
    n670 = local write "L2 Ctrl Loop Out Actuator"(w1533) -> ()
    n671 = local write "L2 Cmd  Volts"(w1526) -> ()
    n672 = local write "L2 Autobalance Out"(w1527) -> ()
    n673 = Wait Until Next ms Multiple(millisecond multiple=u32 4) -> ()  [unwired: 1 out]
  }
  n674 = flat-sequence {
    tunnel: [w1621] -> w73
    tunnel: [w1623] -> w72
    tunnel: [w1622] -> w71
    tunnel: w10 -> [_]
    tunnel: [w1616] -> w61
    frame #0 {
      n675 = global read "Global Cache.vi" "L1 Calibrations"() -> (w1615:T46)
      n676 = Unbundle By Name(w1615) -> ("Command Sensitivity"=w1621:dbl[], "Servo Error Offset"=w1616:dbl[], "LVDT Sensitivity"=w1617:dbl[], "LVDT Offset"=w1620:dbl[], "Load Cell Offsets"=w1619:dbl[], "Load Cell Sensitivity"=w1618:dbl[])
      n677 = Build Array (concatenate)(w1620, w1619) -> (w1623:dbl[])
      n678 = Build Array (concatenate)(w1617, w1618) -> (w1622:dbl[])
    }
  }
  n679 = Initialize Array(0.0 ("element"), 2 ("dimension size"), 6 ("dimension size")) -> (w51:dbl[][])
  n680 = while {
    shift-right: [w1624] -> _
    shift-left: w51 -> [w1635]
    shift-right: [w1629] -> _
    shift-left: w13 -> [w1631]
    tunnel: w96 -> [w1628]
    tunnel: [w1627] -> w87
    stop <- w1627 stop-if-true
    # "Store Previous Command"
    n681 = local read "L1 Ctrl Loop In Actuator"() -> (w1626:dbl[])
    n682 = local read "L2 Ctrl Loop In Actuator"() -> (w1625:dbl[])
    n683 = Build Array(w1626, w1625) -> (w1624:dbl[][])
    n684 = Not Equal?(x=w1624, y=w1635) -> (x != y?=w1634:bool[][])
    n685 = Or Array Elements(Boolean array=w1634) -> (logical OR=w1633:bool)
    n686 = case shown="False" w1633 {
      tunnel: w1624 -> [_ w1645]
      tunnel: w1631 -> [w1637 w1641]
      tunnel: [w1637 w1639] -> w1630
      tunnel: w1628 -> [_ w1638]
      frame False {
      }
      frame True {
        n687 = local read "Logging Directory"() -> (w1648:path)
        n688 = Build Path(base path=w1648, name or relative path=w1638) -> (appended path=w1647:path)
        n689 = Open/Create/Replace File(file path (use dialog)=w1647, error in=w1641, operation (0:open)=T57."replace or create") -> (refnum out=w1644:refnum<file>, error out=w1640:errorcluster)  [unwired: 4 out]
        n690 = Write to Binary File(file (use dialog)=w1644, data=w1645, error in=w1640) -> (refnum out=w1642:refnum<file>, error out=w1643:errorcluster)  [unwired: 4 out]
        n691 = Close File(refnum=w1642, error in=w1643) -> (error out=w1639:errorcluster)  [unwired: 1 out]
      }
    }
    n692 = local read "App Running"() -> (w1636:bool)
    n693 = Wait Until Next ms Multiple(millisecond multiple=u32 2000) -> ()  [unwired: 1 out]
    n694 = call "Error Logger.vi"("error in (no error)"=w1630) -> ("error out"=w1629:errorcluster)  [unwired: 1 in, 9 out]
    n695 = Not(x=w1636) -> (.not. x?=w1627:bool)
  }
  n696 = while {
    shift-right: [w1664] -> _
    shift-left: w10 -> [w1669]
    tunnel: w72 -> [w1668]
    tunnel: w71 -> [w1667]
    tunnel: w66 -> [w1663]
    tunnel: w67 -> [w1662]
    tunnel: [w1656] -> w93
    tunnel: w39 -> [w1654]
    shift-right: [w1651] -> _
    shift-left: w56 -> [w1653]
    tunnel: w57 -> [w1652]
    shift-right: [w1650] -> _
    shift-left: FALSE -> [w1649]
    stop <- w1656 stop-if-true
    # "DAQ Loop"
    n697 = local read "DAQ Enabled"() -> (w1666:bool)
    n698 = case shown="True" w1666 {
      tunnel: w1669 -> [w1680 w1704]
      tunnel: [w1680 w1700] -> w1664
      tunnel: w1668 -> [_ w1703]
      tunnel: w1667 -> [_ w1702]
      tunnel: w1663 -> [_ w1699]
      tunnel: w1662 -> [_ w1698]
      tunnel: [w1679 w1696] -> w1660
      tunnel: [w1676 w1695] -> w1659
      tunnel: [w1672 w1694] -> w1658
      tunnel: [_ TRUE] -> w1657
      tunnel: [w1676 w1691] -> w1655
      tunnel: w1654 -> [_ w1689]
      tunnel: w1653 -> [w1674 w1688]
      tunnel: w1652 -> [_ w1687]
      tunnel: [w1674 w1686] -> w1651
      tunnel: [w1675 w1683] -> w1650
      tunnel: w1649 -> [w1675 w1682]
      frame False {
        w1673 = 2 ("dimension size")
        w1670 = 0.0 ("element")
        w1671 = 6 ("dimension size")
        n699 = Initialize Array(0.0 ("element"), 12 ("dimension size"), w1673) -> (w1676:dbl[][])
        n700 = Initialize Array(w1670, w1671, w1673) -> (w1679:dbl[][])
        n701 = Initialize Array(w1670, w1671) -> (w1672:dbl[])
        n702 = Wait Until Next ms Multiple(millisecond multiple=u32 500) -> ()  [unwired: 1 out]
      }
      frame True {
        n703 = local read "Number of \nExternal \nChannels"() -> (w1701:i32)
        n704 = call "Daq Receive.vi"("Daq Actions"=Daq_Actions."Get Responses", "error in (no error)"=w1704) -> ("Responses"=w1692:dbl[], "error out"=w1685:errorcluster)  [unwired: 1 in, 6 out]
        n705 = case shown="True" w1682 {
          selector: w1682 -> [_ w1715]
          tunnel: w1688 -> [w1711 w1716]
          tunnel: w1687 -> [w1713 _]
          tunnel: [w1710 w1716] -> w1686
          tunnel: w1685 -> [w1709 w1714]
          tunnel: [w1708 w1714] -> w1684
          tunnel: [TRUE w1715] -> w1683
          frame False {
            n706 = Bundle By Name(cluster=w1713, "Command"=Mixed_Mode_Command_Action."Start Acquisition") -> (w1712:T34)
            n707 = Enqueue Element(queue=w1711, element=w1712, error in (no error)=w1709) -> (queue out=w1710:refnum<queue>, error out=w1708:errorcluster)  [unwired: 1 in, 1 out]
          }
          frame True {
          }
        }
        n708 = local write "DAQ Volts"(w1692) -> ()
        n709 = Unbundle By Name(w1685) -> ("status"=w1697:bool)
        n710 = call "Split DAQ Data.vi"("L1 Absolute Offsets"=w1703, "L1 Measured Sensitivities"=w1702, "Number of LBCBs"=w1689, "Responses"=w1692, "L2 Absolute Offsets"=w1698, "L2 Measured Sensitivities"=w1699, "Number of \nExternal \nChannels"=w1701) -> ("Servo Error"=w1696:dbl[][], "LVDT & LC"=w1695:dbl[][], "External Channels"=w1694:dbl[], "Volts LVDT & LC"=w1691:dbl[][])  [unwired: 1 in, 4 out]
        n711 = Wait Until Next ms Multiple(millisecond multiple=u32 2) -> ()  [unwired: 1 out]
        n712 = call <vilib>:"Clear Errors.vi"("error in (no error)"=w1684) -> ("error out"=w1700:errorcluster)  [unwired: 6 out]
        n713 = local write "DAQ Overflow"(w1697) -> ()
      }
    }
    n714 = local write "DAQ Started"(w1657) -> ()
    n715 = local read "App Running"() -> (w1665:bool)
    n716 = local write "Servo Error"(w1660) -> ()
    n717 = local write "Actuator Meas. Disp & Forces"(w1659) -> ()
    n718 = local write "Volts LVDT & LC"(w1655) -> ()
    n719 = call "GetSamplingRate.vi"() -> ("Sampling"=w1661:i32)
    n720 = local write "External Sensors"(w1658) -> ()
    n721 = local write "DAQ Rate"(w1661) -> ()
    n722 = Not(x=w1665) -> (.not. x?=w1656:bool)
  }
  n723 = Obtain Queue(element data type="", error in (no error)=w10) -> (queue out=w77:refnum<queue>, error out=w76:errorcluster)  [unwired: 2 in, 2 out]
  n724 = while {
    shift-right: [w1719] -> _
    shift-left: w77 -> [w1722]
    shift-right: [w1720] -> _
    shift-left: w76 -> [w1721]
    tunnel: [w1717] -> w75
    stop <- w1717 stop-if-true
    # "Archive Voltage Readings"
    n725 = Get Queue Status(queue=w1722, error in (no error)=w1721) -> (queue out=w1725:refnum<queue>, error out=w1726:errorcluster, # elements in queue=w1724:i32)  [unwired: 6 out]
    n726 = Wait Until Next ms Multiple(millisecond multiple=u32 2000) -> ()  [unwired: 1 out]
    n727 = Greater Than 0?(x=w1724) -> (x > 0?=w1723:bool)
    n728 = case shown="True" w1723 {
      tunnel: w1725 -> [w1730 w1739]
      tunnel: w1726 -> [w1729 w1738]
      tunnel: [w1729 w1735] -> w1727
      tunnel: [w1730 w1737] -> w1719
      frame False {
        n729 = Wait Until Next ms Multiple(millisecond multiple=u32 100) -> ()  [unwired: 1 out]
      }
      frame True {
        n730 = Flush Queue(queue=w1739, error in (no error)=w1738) -> (queue out=w1737:refnum<queue>, remaining elements=w1736:string[], error out=w1733:errorcluster)
        n731 = Concatenate Strings(w1736) -> (w1734:string)
        n732 = call "Save Text Data.vi"("String"=w1734, "LogFile Type"=LogFileType."Volts", "error in"=w1733) -> ("error out"=w1735:errorcluster)  [unwired: 2 in, 1 out]
      }
    }
    n733 = local read "App Running"() -> (w1728:bool)
    n734 = Not(x=w1728) -> (.not. x?=w1717:bool)
    n735 = call "Error Logger.vi"("error in (no error)"=w1727) -> ("error out"=w1720:errorcluster)  [unwired: 1 in, 9 out]
  }
  n736 = while {
    shift-right: [w1742] -> _
    shift-left: w77 -> [w1744]
    shift-right: [w1741] -> _
    shift-left: w76 -> [w1743]
    tunnel: [w1740] -> w74
    stop <- w1740 stop-if-true
    # "Collect Voltage Readings"
    n737 = call "App Status Globals.vi"("App Status Actions"=App_Status_Actions."Get Status") -> ("App Status Out"=w1748:T52)  [unwired: 5 in, 9 out]
    n738 = Unbundle By Name(w1748) -> ("Voltage Logging"=w1746:bool)
    n739 = local read "Volt Logger Time"() -> (w1745:u32)
    n740 = case shown="True" w1746 {
      tunnel: w1744 -> [w1751 w1756]
      tunnel: w1743 -> [w1750 w1755]
      tunnel: [w1751 w1753] -> w1742
      tunnel: [w1750 w1752] -> w1741
      frame False {
      }
      frame True {
        n741 = local read "L1 Cmd  Volts"() -> (w1760:dbl[])
        n742 = local read "L2 Cmd  Volts"() -> (w1759:dbl[])
        n743 = local read "DAQ Volts"() -> (w1758:dbl[])
        n744 = Build Array (concatenate)(w1760, w1759, w1758) -> (w1757:dbl[])
        n745 = call "Data 2 Record.vi"("Data"=w1757) -> ("Records"=w1754:string)  [unwired: 2 in, 8 out]
        n746 = Enqueue Element(queue=w1756, element=w1754, error in (no error)=w1755) -> (queue out=w1753:refnum<queue>, error out=w1752:errorcluster)  [unwired: 2 out]
      }
    }
    n747 = Wait Until Next ms Multiple(millisecond multiple=w1745) -> ()  [unwired: 1 out]
    n748 = local read "App Running"() -> (w1749:bool)
    n749 = Not(x=w1749) -> (.not. x?=w1740:bool)
  }
  n750 = Obtain Notifier(name (unnamed)="Command & Stiffness Changes", notification data type=w7, error in (no error)=w10) -> (notifier out=w6:refnum<notifier>, error out=w8:errorcluster)  [unwired: 1 in, 1 out]
  n751 = while {
    shift-right: [w1768] -> _
    shift-left: w9 -> [w1772]
    tunnel: w7 -> [w1766]
    shift-right: [w1764] -> _
    shift-left: w6 -> [w1765]
    shift-right: [w1762] -> _
    shift-left: w8 -> [w1771]
    tunnel: [w1761] -> w5
    stop <- w1761 stop-if-true
    n752 = Dequeue Element(queue=w1772, timeout in ms (-1)=2000, error in (no error)=w1771) -> (queue out=w1768:refnum<queue>, element=w1767:T26, timed out?=w1769:bool, error out=w1763:errorcluster)
    n753 = case shown="False" w1769 {
      tunnel: w1767 -> [w1774 _]
      tunnel: w1766 -> [w1779 _]
      tunnel: w1765 -> [w1778 w1805]
      tunnel: [w1777 w1805] -> w1764
      tunnel: w1763 -> [w1776 w1804]
      tunnel: [w1775 w1804] -> w1762
      frame False {
        n754 = case shown="\"Iterative Command Update\"" w1774 {
          selector: w1774 -> [w1785 w1793 w1801]
          tunnel: w1779 -> [w1787 w1795 w1803]
          tunnel: w1778 -> [w1784 w1792 w1800]
          tunnel: [w1783 w1791 w1799] -> w1777
          tunnel: w1776 -> [w1782 w1790 w1798]
          tunnel: [w1781 w1789 w1797] -> w1775
          frame "Stiffness Update" {
            n755 = local read "Stiffness Jacobian Column"() -> (w1786:T3[])
            n756 = Bundle By Name(cluster=w1787, "Command || Stiffness Update"=w1785, "Stiffness"=w1786) -> (w1780:T25)
            n757 = Send Notification(notification=w1780, notifier=w1784, error in (no error)=w1782) -> (notifier out=w1783:refnum<notifier>, error out=w1781:errorcluster)
          }
          frame "Command Update" {
            n758 = local read "Current Target"() -> (w1794:T5[])
            n759 = Bundle By Name(cluster=w1795, "Command || Stiffness Update"=w1793, "Target"=w1794) -> (w1788:T25)
            n760 = Send Notification(notification=w1788, notifier=w1792, error in (no error)=w1790) -> (notifier out=w1791:refnum<notifier>, error out=w1789:errorcluster)
          }
          frame "Iterative Command Update" {
            n761 = local read "Iterative Target"() -> (w1802:T5[])
            n762 = Bundle By Name(cluster=w1803, "Command || Stiffness Update"=w1801, "Target"=w1802) -> (w1796:T25)
            n763 = Send Notification(notification=w1796, notifier=w1800, error in (no error)=w1798) -> (notifier out=w1799:refnum<notifier>, error out=w1797:errorcluster)
          }
        }
      }
      frame True {
      }
    }
    n764 = local read "App Running"() -> (w1773:bool)
    n765 = Not(x=w1773) -> (.not. x?=w1761:bool)
  }
  n766 = Compound Arithmetic op=AND(w87, w93, w92, w91, w90, w89, w88, w5, w75, w74) -> (w86:bool)
  n767 = flat-sequence {
    tunnel: w86 -> [w1808]
    frame #0 {
      n768 = local write "All Stopped"(w1808) -> ()
      n769 = call "NoArgumentsLauncher.vi"("Application"=NoPanelAppTypes."Control Loops", "Application Launcher Actions"=Launcher_Actions."Stop") -> ()  [unwired: 1 in, 9 out]
    }
  }
